vi "DAQ_Output TF.vi"(0 "System DAQ params to use:":u16(ring)=6 items=["MPS Rx", "MPS Tx", "Human Tx", "Rodent Tx", "Rodent Tx coupling (VRx)", "Rodent Rx", "Human Rx", "Manual Input"], 1 "TF_Params":T3={"Start freq (Hz)"=1000.0, "Stop freq (Hz)"=500000.0, "delta f (Hz)"=50.0, "samples per channel"=50000, "fsamp (Hz)"=2000000.0, "downsampling factor"=1.0, "Attenuation factor"=1.0} {"Start freq (Hz)" format="%#_6p"; "Stop freq (Hz)" format="%#_6p"; "delta f (Hz)" format="%#_6p"; "samples per channel" format="%.0p"; "fsamp (Hz)" format="%#_6p"; "downsampling factor" format="%#_6p"; "Attenuation factor" format="%#_6p"}, 2 "Save File?":bool=TRUE, 3 "string append to saved name":string="MPS_Tx_WithIMonNotch", 5 "Rogowski Scaling?":bool, 7 "Techron Gain Scaling":bool, 9 "Preamp Gain":dbl=1.0, 12 "User define frequency?":bool, 13 "Output all user defined value":bool, 14 "user defined \noutput value":dbl=0.1) -> (4 "TF mag output":dbl[](array[numeric])=[2.0372154916289125e-07, 6.793559181104437e-07, 1.696335790070309e-06, 2.1296488090751283e-06, 1.0109049448492243e-06, 3.242527142614195e-07, 2.01786175812527e-06, 1.3716083741435276e-06, 1.8749207637441033e-07, 5.690020511841858e-07, 1.3831526970474158e-06, 9.031002498074619e-07, 2.3120965479170196e-07, 4.2637533270188516e-07, 1.2717129807954672e-06, 6.739401216156862e-07, 9.502797117923468e-07, 1.4761926503177053e-06, 4.2449444146675436e-07, 1.3766268206166872e-06, 1.1574135065424225e-06, 4.390152066215787e-07, 1.4693364715610942e-07, 9.277841552509502e-07, 2.5102632307106685e-07, 1.5213042828718781e-06, 1.628993469736173e-06, 7.546981171721333e-07, 1.0427860563616102e-06, 9.714940189259299e-07, 1.43702270277105e-06, 1.2400316803756997e-06, 1.0637541376139376e-06, 7.466040945341502e-07, 8.974006467013478e-07, 3.6902682451535563e-07, 1.1637652293582506e-06, 6.6529859461445e-07, 1.5372963939506228e-06, 1.0372235089020587e-06, 1.3395277070635045e-06, 1.0361944250161835e-06, 1.3508414174132359e-06, 1.3622047310919937e-06, 1.0919652013386314e-06, 3.574766379241672e-07, 1.1659572050191398e-06, 6.189314025390137e-07, 1.0807867648715636e-07, 1.5380539400614782e-06, 1.6263735527414179e-06, 5.32112681526953e-07, 1.4310309890370497e-06, 1.4351885732615034e-06, 8.584318672907275e-07, 1.12233373437069e-06, 4.815228840574134e-07, 5.411977015167934e-07, 1.4144329557252704e-06, 1.1497955449729725e-06, 1.1095408290289881e-06, 9.59365615054982e-07, 1.8710766553428788e-06, 4.100069077682547e-07, 2.0252669578614933e-06, 2.0691205927940387e-06, 1.8891821441695545e-06, 2.0084794530702413e-06, 1.011117507818362e-06, 7.380670323609788e-07, 1.6387142491343077e-06, 9.327501315313441e-07, 1.8591321524715755e-06, 1.4227070668243068e-06, 2.6885456636705938e-06, 1.734732141488192e-06, 1.5359992596700657e-06, 2.9417755244459883e-06, 1.7998117427665506e-06, 1.2302735256347795e-06, 2.2271101093460748e-06, 2.0734509814401154e-06, 2.4002547859215057e-06, 1.4539712262088093e-06, 4.7436064752972777e-07, 1.882518473346791e-06, 2.9825459503646984e-06, 1.341447255240376e-06, 3.1473647714171137e-06, 2.401999152339036e-06, 3.830836392519218e-06, 2.7205751977305096e-06, 2.8678776825669147e-06, 3.3763181271312693e-06, 2.238606088769139e-06, 2.8006224623551447e-06, 4.226545237517427e-06, 3.936317527625128e-06, 3.5126357457397537e-06, 4.293951113248438e-06, 3.822800804203132e-06, 4.5225707303408105e-06, 4.0434439252313434e-06, 4.854193842370676e-06, 5.451288943225746e-06, 4.44612502569016e-06, 4.866573414449756e-06, 5.675666006001769e-06, 5.4403891145442125e-06, 5.75961684673854e-06, 4.870583216911151e-06, 6.4256941483989454e-06, 7.723671846367389e-06, 7.4837204474723845e-06, 6.222218548855555e-06, 7.590438086205701e-06, 7.5188758620780854e-06, 8.521498643916568e-06, 6.249152687634874e-06, 7.566289155689773e-06, 9.745623816846875e-06, 9.758296789658542e-06, 8.890595348675359e-06, 8.931120791337168e-06, 1.0399248680151127e-05, 1.0838503336982061e-05, 1.1260685540728752e-05, 1.082378468051051e-05, 1.2806779207580574e-05, 1.114960676394728e-05, 1.257128261917567e-05, 1.5416848441356857e-05, 1.4683523018574373e-05, 1.2611982709294083e-05, 1.642105662766135e-05, 1.5922423733550202e-05, 1.491421790154185e-05, 1.5578341427846582e-05, 1.659821358399733e-05, 1.709785681614034e-05, 1.8945273766490233e-05, 1.9363359923778153e-05, 1.9502597442375368e-05, 2.0639570485776163e-05, 2.0543207769782197e-05, 2.1691234755881526e-05, 2.2267028376064175e-05, 2.329089681548961e-05, 2.264594187261997e-05, 2.495996330527915e-05, 2.6105168892792582e-05, 2.7135537446387392e-05, 2.666988817069712e-05, 2.858416752662035e-05, 2.942859399006933e-05, 3.206928489966959e-05, 3.223048627196298e-05, 3.328739308435493e-05, 3.52415347598883e-05, 3.625643354079973e-05, 3.6778519243786124e-05, 3.811910848670486e-05, 3.90858476210099e-05, 4.221004792496587e-05, 4.22374549045834e-05, 4.5537077660884215e-05, 4.6308159049720095e-05, 4.878439550948665e-05, 4.9595461365732126e-05, 5.0734266319742015e-05, 5.335814071346675e-05, 5.617936948647044e-05, 5.7503826421850815e-05, 5.897541384195838e-05, 6.172515297231758e-05, 6.443664154470796e-05, 6.668646219152251e-05, 6.888677020126689e-05, 7.212234401398264e-05, 7.4933870118391e-05, 7.851452682634401e-05, 7.885553502658508e-05, 8.224084112024173e-05, 8.729351248339771e-05, 8.906874761983332e-05, 9.236254808123519e-05, 9.768310963065837e-05, 9.993873715919868e-05, 0.00010339897754066812, 0.00010898173400692462, 0.00011160171243173072, 0.00011706398053056314, 0.00012127098890446096, 0.00012650149142309162, 0.00013171434236989966, 0.00013758405099720852, 0.00014324117473233077, 0.00014863093132722968, 0.00015594197945553, 0.0001619041881869678, 0.00016946556001067674, 0.0001761666805086842, 0.00018437709377742338, 0.00019080859604449582, 0.00019887675407958386, 0.00020802928325185506, 0.00021735351743626773, 0.00022759683965656942, 0.00023772990243054828, 0.00024814096047077235, 0.0002577463712794448, 0.00026986599649594684, 0.00028340467395312254, 0.0002948052391906649, 0.00031149643710847764, 0.00032422266286623764, 0.00034155758920128947, 0.0003580001722440461, 0.00037535168678973295, 0.00039409138977495846, 0.00041430294696878433, 0.00043639323383142274, 0.0004607030690792594, 0.00048437378201234195, 0.0005116261720156887, 0.0005392744247378722, 0.0005716075743237706, 0.0006036990023538168, 0.0006382950959561843, 0.0006768368311226179, 0.0007184789659525549, 0.0007623862947976867, 0.0008130285347634719, 0.000865328852128615, 0.0009239292602682656, 0.0009882489296444742, 0.0010568390476129361, 0.0011338393422531956, 0.0012183921127213921, 0.0013138792442572388, 0.001418003747640743, 0.001535522947424366, 0.0016664493156874076, 0.001813297378252482, 0.0019799233643365286, 0.0021645534102197957, 0.0023784902298449747, 0.0026162768861308955, 0.002889733654480595, 0.0031963722989208, 0.0035374011016199606, 0.003914657200955006, 0.004323004729336459, 0.004753851195795146, 0.0051904836504763855, 0.005609851465877228, 0.005981794396312844, 0.006261726821948118, 0.00641179468539871, 0.006402195594109291, 0.006244408095304624, 0.00598702098189062, 0.005684764211770975, 0.005378027040291605, 0.005088639918349321, 0.004824671537009969, 0.004594773179979079, 0.004388250540076509, 0.0042074314116050835, 0.0040484671810071945, 0.003910154547206496, 0.0037847184253491078, 0.003676490229089884, 0.0035809616298052935, 0.0034950133528669955, 0.003419160313056956, 0.003355105939834968, 0.0032971154760109383, 0.0032458309179729584, 0.0032037401790805022, 0.003164161771550465, 0.0031327328175114557, 0.0031091482035021877, 0.003085498228113483, 0.0030690459185469996, 0.0030568044311039865, 0.0030461709143044836, 0.003041197505528879, 0.003041706349357348, 0.0030435455495283863, 0.0030495319370752966, 0.003057692641077951, 0.0030704250999599473, 0.0030849256090688644, 0.0031043793588513427, 0.0031261014737604203, 0.0031491108517110703, 0.0031771001385535913, 0.0032073608053417384, 0.0032436774293707585, 0.003279813325587537, 0.0033208704142117305, 0.0033637626362167028, 0.0034091342630075505, 0.0034592404274854695, 0.00351448277784265, 0.0035727253361016384, 0.0036334133511267274, 0.0036966059085619266, 0.003767518173210152, 0.0038413323284179116, 0.0039178981357463425, 0.004000713688535257, 0.004086254616971957, 0.0041774025214381645, 0.004274692122950266, 0.004374586450587849, 0.004480428652522378, 0.004592336922758399, 0.0047063586220150435, 0.004828329315829819, 0.004952304484767822, 0.005083864418425228, 0.005219992544257958, 0.005360572150230163, 0.005503310775577753, 0.005650178099919648, 0.005797876043917457, 0.005947310317132557, 0.00609322438643053, 0.006240068116715204, 0.006381286601970306, 0.0065199452791355975, 0.006648805426228001, 0.006764667255400801, 0.00687148605986856, 0.0069620532378664385, 0.007034500737286003, 0.007088490320480461, 0.007123016978728839, 0.007135629768528894, 0.0071272667489462455, 0.007097935162051244, 0.00704688833896544, 0.00698063251987629, 0.0068993456960810325, 0.0068020652511235295, 0.006690301151635434, 0.006572939495142656, 0.006445477583369852, 0.006313942018104493, 0.006176322525557588, 0.006042932950458157, 0.0059062422568806885, 0.005759142682368877, 0.005619395191586785, 0.005500699809907893, 0.0053677371581780774, 0.005240933031342609, 0.005116506843688415, 0.004997998143370529, 0.004882573974520269, 0.0047699918897461824, 0.0046653540271694065, 0.00456423216909828, 0.004465264326574151, 0.004374492456427474, 0.004285528727967664, 0.004199866013002946, 0.004117968553655641, 0.004042080261713175, 0.0039676189128161595, 0.0038954429953121715, 0.003829986170977068, 0.0037660919612099294, 0.0037041343225806614, 0.0036459363198869895, 0.003590625647267971, 0.0035373602829234093, 0.0034856488342473882, 0.0034397914012131714, 0.0033936480297744203, 0.003349844232891371, 0.0033070063257520676, 0.003270540153728508, 0.003232013758206085, 0.0031971683916848528, 0.003164100942299467, 0.003132074968409261, 0.003102906016181999, 0.0030749530093250694, 0.003048557411793342, 0.0030251150856024337, 0.003001299830241231, 0.0029798512534916447, 0.0029588722539942622, 0.0029426250122048113, 0.0029261826415382143, 0.0029099037261367143, 0.002897980720198404, 0.00288340882160916, 0.002874341499206318, 0.0028661737074489224, 0.002857012307988124, 0.0028517467867249452, 0.002849270969549165, 0.0028426491181320385, 0.002843598198764933, 0.0028456501701090817, 0.002846987016539148, 0.0028546148348877858, 0.002861468125705527, 0.0028696341944694655, 0.0028821643213220263, 0.0028958483242476148, 0.0029124092621891392, 0.002932028600726075, 0.002955969060847836, 0.0029808809710248755, 0.00301074312654329, 0.003044911212316796, 0.003086668441052093, 0.003123561677421555, 0.003177631079607654, 0.003220900345320899, 0.003283404786445936, 0.0033335077077304505, 0.003415158770545732, 0.0034917469944288613, 0.003574823389508343, 0.0036591756984979628, 0.0037449425633328494, 0.0038316979794502395, 0.003908487950184218, 0.003968842309478478, 0.004003554932827288, 0.004000305003242141, 0.003944326724562689, 0.0038282707078578357, 0.0036551095435839055, 0.003430591002762993, 0.0031729199038966985, 0.002897570133363583, 0.0026221348457451253, 0.0023620070095678857, 6.164614697188743e-07, 0.0019030029843609476, 0.0017124606132191383, 0.0015463391035798878, 0.0014045425244661302, 0.001283156041583334, 0.0011783872907193238, 0.0011062852186959325, 0.0010345130604953571, 0.0009862645351283305, 0.000951913213045555, 0.000930822971927366, 0.0009229063773060129, 0.0009278401171160928, 0.000947666169095748, 0.0009782281520481502, 0.0010238234384319386, 0.0010867909292265497, 0.0011655078777641108, 0.0012626822383428405, 0.0013807053346902112, 0.001518885518425445, 0.0016807681781777079, 0.0018709546877245882, 0.0020858300920659273, 0.002328247444811447, 0.0025927272793475984, 0.0028785096374129744, 0.0031688479973878093, 0.003448477146808804, 0.003703943351999831, 0.003916319650435753, 0.004072372564256995, 0.004174102273354721, 0.004222381703749427, 0.004228257581942058, 0.004198666137537497, 0.004150743924274754, 0.004089118026205858, 0.00402012832415787, 0.003953650143401563, 0.0038847672330356367, 0.003820782968838551, 0.0037626870141772508, 0.003705343736908736, 0.003658006130046551, 0.003614856738190562, 0.0035784208320527515, 0.0035434238584049283, 0.003514160478534067, 0.003488170700812893, 0.003468622707332244, 0.003443915344896603, 0.0034314299162463134, 0.0034246630437881663, 0.003416544978817137, 0.0034119641099697425, 0.0034088364558863206, 0.0034083014897694965, 0.0034117155961883717, 0.0034159402473708006, 0.0034217779007516633, 0.003430072444593314, 0.003440049913353305, 0.0034538917831024966, 0.0034669055423229133, 0.0034833364863646864, 0.003501628475332639, 0.0035196197032543912, 0.003540336254543647, 0.0035622786880641732, 0.003585694628045036, 0.003611895491815887, 0.003640008384025932, 0.003667157114489658, 0.003696788673689253, 0.0037309122101256507, 0.003762746847704778, 0.0037970057968524425, 0.0038353516289641766, 0.0038714577040932846, 0.0039113841049076715, 0.00395147652947973, 0.003995491778150964, 0.00403812158458586, 0.004087585217075255, 0.004134714990345707, 0.004184749090863663, 0.004237536259964986, 0.004289462606464673, 0.004345586835427315, 0.004404102710112459, 0.004463315212311432, 0.004525851738043004, 0.004588374389625155, 0.004657469223876116, 0.00472500859303859, 0.0047969494885303195, 0.00487141632955198, 0.004947756733803814, 0.005026829427225351, 0.005108658634518159, 0.005194617350463291, 0.00528248025974792, 0.005371866803911184, 0.005466752222299172, 0.005562387013028619, 0.00566560323632966, 0.005767577425601827, 0.00587687501776066, 0.005987009019026231, 0.006102088996437571, 0.006223627687271268, 0.006345229034043439, 0.00647128049002447, 0.006605011436205142, 0.006739802231268402, 0.0068799279793823566, 0.007024819960270474, 0.0071753374378373215, 0.007327972898878207, 0.0074888643285302555, 0.0076499912263523805, 0.00781978907948591, 0.007994419869134756, 0.00817024970975524, 0.008349410641485283, 0.008535727849152727, 0.008723027999915828, 0.008916179810292683, 0.009110973170224202, 0.009310867548075983, 0.00951180121726737, 0.009711672504489894, 0.009913334696390445, 0.010112796222984012, 0.01031388040365655, 0.010512437920119903, 0.010704567828247245, 0.010895515977437925, 0.011074623324110815, 0.011248750272778663, 0.011411509034678248, 0.011562649968872745, 0.011701942061589638, 0.011832798950041565, 0.011940517202510381, 0.012037413785487755, 0.012114521830438083, 0.012174924860481079, 0.012216767323894755, 0.012243209207602959, 0.012247709617285987, 0.012240010247821648, 0.012209836313097716, 0.012168028995498176, 0.012109759173068004, 0.012034522182703776, 0.011948772525407365, 0.011851525989082679, 0.011745454590657902, 0.011628240665402894, 0.011505038496599857, 0.011376852844174962, 0.011239735443193379, 0.011103832677707079, 0.010962850555773767, 0.010822065607391079, 0.010680625672971084, 0.010535385013054266, 0.01039054769482169, 0.01025176171211727, 0.010113251395753366, 0.009971691355567611, 0.009834262067813083, 0.009702255710372124, 0.009574029455887891, 0.009446822900503322, 0.009319720522908803, 0.009201529228534809, 0.009082694467120624, 0.008971962377477155, 0.008861154816449937, 0.008756517789594447, 0.008653410153402935, 0.00855409504766486, 0.008457961508651883, 0.008367952582596505, 0.008278244688673891, 0.008192999415495356, 0.008111552392976442, 0.008036794780504616, 0.00796144879230125, 0.007888979685585542, 0.007819344480339802, 0.007754288285094333, 0.007694339832065249, 0.007634104724108179, 0.007575291221359333, 0.007522567947202587, 0.007469221398234218, 0.007423758302493742, 0.007378140377463572, 0.007335127075570248, 0.007292968067296177, 0.007259098778388161, 0.007222119021201777, 0.007190322865531502, 0.007160372613883688, 0.0071328789176969744, 0.007106856861104297, 0.007086815067238445, 0.007065491821345224, 5.546838338613242e-07, 0.007031486378227067, 0.007019384683356254, 0.007010062760928216, 0.007000077530297156, 0.006995370883301304, 0.006991647291921397, 0.006990644822433608, 0.006991325452510118, 0.006995689108552698, 0.0070002833959157745, 0.007008318610279569, 0.007021193674572225, 0.007032760654437141, 0.00704952640215466, 0.007068003637619281, 0.007090315730289243, 0.007111636934614471, 0.007141592610911906, 0.0071683670064617636, 0.007201021141207065, 0.007236459974853032, 0.007277386141220549, 0.007316987402201348, 0.007363517240918104, 0.007409807563783298, 0.007462479587681477, 0.007518549491041108, 0.007576989843540695, 0.007636498399831262, 0.007705430767937352, 0.007778317588309633, 0.007852434050960916, 0.007929901774595809, 0.008015542942976071, 0.008103912510163734, 0.008200019508343339, 0.008296823702025974, 0.008406222769244142, 0.008514706615279491, 0.008636830705876924, 0.008758847294239562, 0.008894024140768399, 0.009032297369439196, 0.009181338441392796, 0.009326957459033012, 0.009501365304138455, 0.009674120938744847, 0.009859894704024064, 0.010053693985701787, 0.010259551491084148, 0.010479289260633656, 0.010707560752033028, 0.01095149664420516, 0.011210562391792548, 0.011486347046830546, 0.01177137799579019, 0.012073752819968331, 0.012395791965619964, 0.012729353691860342, 0.013089748942432861, 0.013460368571250637, 0.01385977342398694, 0.014265912195477652, 0.014697306686528744, 0.01514034539102792, 0.01560757849564455, 0.016075815847262413, 0.016564786538784054, 0.01704467463433095, 0.017533088951704023, 0.018015748889576716, 0.018475590459784356, 0.01889974690987198, 0.01930318427234332, 0.01964640577240411, 0.019925382568646396, 0.020228750568243768, 0.020265656705801476, 0.020297101520647225, 0.02024819226764239, 0.020098609687792555, 0.019856752080114056, 0.01953181759374221, 0.019144129055940963, 0.01867901461616855, 0.018180542030335513, 0.017641175407968206, 0.017085042585021932, 0.01651585903499849, 0.015949546801429192, 0.015382417645858707, 0.014834707677971133, 0.014296118869649967, 0.013782714967972598, 0.013282214801240469, 0.012811679509594128, 0.01235581070612155, 0.011927878790376219, 0.011519248800922687, 0.011127343542270155, 0.010752867280692132, 0.010411375755346888, 0.010078041405944737, 0.009767792276147947, 0.00947034287789845, 0.009191394000659462, 0.008924938111006048, 0.00867416964508942, 0.008435748159650501, 0.008211731744829516, 0.00799628612106185, 0.007798892356861463, 0.007602257981305233, 0.007423579551743067, 0.007249260954099596, 0.007087197639072701, 0.006930931211151319, 0.006786447695694304, 0.006643871181243099, 0.006511490766310069, 0.006385141774894306, 0.006267532596712949, 0.0061546566403550725, 0.006047018999790388, 0.005941378993852128, 0.00584868739064578, 0.0057546480814531795, 0.005667347668829675, 0.005586641463647396, 0.005508203587509282, 0.005433859524928404, 0.0053663009906424666, 0.005303500780531138, 0.005237420541909372, 0.0051812790486258035, 0.005127022459714558, 0.005075951477162811, 0.005030904536023909, 0.004986705805615258, 0.0049495604105589345, 0.004911452237008161, 0.004878000151050528, 0.004848643960764925, 0.004820642274108188, 0.004798972787378096, 0.004778082269931038, 0.00476188171304398, 0.004747220842243101, 0.0047354648145581085, 0.004727605176166839, 0.0047231266040788575, 0.004723463322165673, 0.0047234203044524145, 0.004729862440449979, 0.004738910028400524, 0.004751708118108957, 0.00476396834240096, 0.0047829184196307205, 0.004804059455298296, 0.004826942512691633, 0.004854623108493706, 0.004883439403248536, 0.004918143878170193, 0.004951495940519052, 0.004986553952624207, 0.005024245245054637, 0.005062482316529173, 0.005096471034425928, 0.005128313819767421, 0.005160779122739624, 0.005187588441927762, 0.00520399372392812, 0.005211739706816874, 0.005209051196474495, 0.005194689792525376, 0.005162054410679822, 0.005113774627149544, 0.005046082674903037, 0.004959945257122816, 0.0048543749246190955, 0.0047262901579443175, 0.004588743282303231, 0.004433977168555782, 0.004267307407971839, 0.004090938607897501, 0.00391167568652165, 0.003728920388539005, 0.003543671676833687, 0.0033621656039902314, 0.0031853263396406034, 0.00301245296775813, 0.0028467892137657045, 0.0026879681915949784, 0.002537911379031695, 0.0023958245784159106, 0.0022605598807129506, 0.002131527399077782, 0.002013108429582286, 0.0018994132677840946, 0.0017943346889407246, 0.0016936111510475094, 0.001600469525632794, 0.0015115940886708712, 0.0014304339331459414, 0.001353339985544366, 0.0012777062666591889, 0.0012195131974909242, 0.0011379246097210683, 0.0010883136080910775, 0.0010313189156855105, 0.0009771522811846648, 0.0009286224642889719, 0.0008808977562469889, 0.0008359982858023881, 0.0007947717424571735, 0.0007548929610178948, 0.000717501683787555, 0.000681324549907791, 0.0006467839458602313, 0.0006200034438237885, 0.0005883191937759186, 0.0005601993506408708, 0.0005313376620691447, 0.0005063887690977925, 0.00048202868815941505, 0.00045916625487411763, 0.00043809039057423347, 0.0004167681990561311, 0.0003972543806660549, 0.0003783056441678319, 0.00036183135494363103, 0.0003438086130131863, 0.0003285076928817975, 0.0003135112552121596, 0.00029902740610936624, 0.000285022946143483, 0.0002717845781508606, 0.00025846023178235006, 0.00024778789406428167, 0.00023657754203818424, 0.00022332645406769833, 0.0002130844148469932, 0.00020518906409604145, 0.00019495229220741514, 0.0001868515457089178, 0.00017666430828974322, 0.00016945486922525382, 0.00016173597016781155, 0.00015427290194259987, 0.00014583017928042558, 0.0001394532040387906, 0.0001324241771500869, 0.0001280933345118669, 0.00012156619509743325, 0.00011824407941880821, 0.00011236776242865911, 0.00010624416956535214, 0.0001027357132786282, 9.92123558802412e-05, 9.197764102919613e-05, 8.931515920821514e-05, 8.719661434611681e-05, 8.244250929818397e-05, 7.94297083637959e-05, 7.813929467799097e-05, 7.603798394004373e-05, 7.350762399698821e-05, 7.12151393165494e-05, 6.895482838131393e-05, 6.671046611850901e-05, 6.407147910490223e-05, 6.389699746887125e-05, 6.247957839954287e-05, 6.289629989829454e-05, 6.194387743455696e-05, 6.135465502450149e-05, 6.087816993385767e-05, 5.816000315461685e-05, 5.923397859448671e-05, 5.86711645637256e-05, 5.863345428538828e-05, 6.070839663391591e-05, 6.0338799568149135e-05, 6.015464172175751e-05, 5.9917620265870535e-05, 5.959781431737995e-05, 6.0454716706029717e-05, 6.063455580839131e-05, 6.009608800981641e-05, 6.387706217422418e-05, 6.34600791090772e-05, 6.431548066813142e-05, 6.457014794584466e-05, 6.593560505304135e-05, 6.4601604384995e-05, 6.63249236881072e-05, 6.604359174471053e-05, 6.675061933962089e-05, 6.713102039404873e-05, 6.681963999985778e-05, 6.768736972693942e-05, 6.9183790534655e-05, 6.942822624230465e-05, 6.982843956190732e-05, 7.193672496854038e-05, 7.021436074452037e-05, 7.17975311597413e-05, 7.183611942498269e-05, 7.012259519525509e-05, 7.377322279735478e-05, 7.29699143899538e-05, 7.204364394322717e-05, 7.43419969560943e-05, 7.469514547335262e-05, 7.474792352170519e-05, 7.535147016489018e-05, 7.588840885577198e-05, 7.640960372794765e-05, 7.489888720309596e-05, 7.603121348222829e-05, 7.723520923735244e-05, 7.716898340179197e-05, 7.879828943663293e-05, 7.878918964207931e-05, 7.839321345408815e-05, 8.067898332242799e-05, 8.023573677573643e-05, 7.933387960652674e-05, 7.879289310481334e-05, 8.083210121646043e-05, 7.918232639055638e-05, 8.120955801247514e-05, 7.963947724208541e-05, 8.232498935875233e-05, 8.05674053536353e-05, 8.18622968308476e-05, 8.207496156961378e-05, 8.15947348367063e-05, 8.124371368542347e-05, 8.220147361838506e-05, 8.33574764778626e-05, 8.242382265869806e-05, 8.365398123681995e-05, 8.293297779392434e-05, 8.439847730918912e-05, 8.368439680869435e-05, 8.363405707304298e-05, 8.384303639641865e-05, 8.422979774229118e-05, 8.364030257485974e-05, 8.403107482227207e-05, 8.367083835093945e-05, 8.41160485051156e-05, 8.531238157073731e-05, 8.508144025133058e-05, 8.590405766901755e-05, 8.477426803288628e-05, 8.543434513154186e-05, 8.533576780752976e-05, 8.659463549318744e-05, 8.535511698671412e-05, 8.613472455143942e-05, 8.490919102595647e-05, 8.625111789073192e-05, 8.635640454191086e-05, 8.698594769204356e-05, 8.6389368874127e-05, 8.61667281379288e-05, 8.64699495096001e-05, 8.595826222889964e-05, 8.723248182699668e-05, 8.64711328992852e-05, 8.693144214833651e-05, 8.683641652517674e-05, 8.78958393738193e-05, 8.734492345960697e-05, 8.783916049823444e-05, 8.61747002264401e-05, 8.768501804301456e-05, 8.714337518653518e-05, 8.747270502178725e-05, 8.750948775232275e-05, 8.74785819433097e-05, 8.792969324249523e-05, 8.73497058898647e-05, 8.930668794129315e-05, 8.779903464005035e-05, 8.828630900858057e-05, 8.889849288226898e-05, 8.855524954678201e-05, 8.964311602247672e-05, 8.810725925489338e-05, 8.962789018095396e-05, 9.014890836021389e-05, 8.915746994358566e-05, 8.930245017529432e-05, 8.878742269477327e-05, 8.940407714523939e-05, 8.968701613923263e-05, 9.088473137324469e-05, 9.027823306624076e-05, 8.977618841059141e-05, 9.012271611846928e-05, 9.057658169548787e-05, 9.15894221167761e-05, 9.028928117230089e-05, 9.063918569159491e-05, 9.25414067258851e-05, 9.298417304110964e-05, 9.134810452844022e-05, 9.190862191879943e-05, 9.339926616916888e-05, 9.212173087654502e-05, 9.246865273698261e-05, 9.306556468780206e-05, 9.303785247470485e-05, 9.277106558924882e-05, 9.192346456547312e-05, 9.262687474891765e-05, 9.330804877002039e-05, 9.30915387511946e-05, 9.38819292239803e-05, 9.543702349636271e-05, 9.560762127592522e-05, 9.508206330111681e-05, 9.5773149779388e-05, 9.608461691968223e-05, 9.731825843248855e-05, 9.537184511560309e-05, 9.54180350620616e-05, 9.679352690109114e-05, 9.732014345971237e-05, 9.813862006561962e-05, 9.775702394087522e-05, 9.849364337657339e-05, 9.829811450182467e-05, 0.00010056198340261321, 9.948285592328476e-05, 0.0001012267969665088, 0.00010026707751442345, 0.00010103461637476879, 0.0001019729753169905, 0.0001023362558214886, 0.00010247887907697833, 0.00010374506914512854, 0.00010197042681756403, 0.00010476583496666581, 0.00010325909274254808, 0.00010629689913288521, 0.00010782386048494457, 0.00010741281145145474, 0.00010785649671445314, 0.00010796738992431124, 0.00010777079182075159, 0.00010921659144371598, 0.00010943866598092394, 0.00011146174333304786, 0.00011084242318885517, 0.00011197824630743252, 0.00011340437595824194, 0.00011272829548002021, 0.00011505593396547745, 0.00011541774570122776, 0.00011616030536194512, 0.00011929865636628787, 0.00011825591447429914, 0.00011955326898795407, 0.00011995860152418436, 0.00012092833277953469, 0.00012270402817089008, 0.00012425441117186207, 0.0001245517907204726, 0.00012645246589899697, 0.00012797859413697687, 0.00012933765190669097, 0.00013037304046320918, 0.00013189593423435948, 0.00013374897228205984, 0.00013426913231691468, 0.00013686423148932193, 0.00013880149350947122, 0.00014026492531460285, 0.00014126619942793188, 0.00014469672761256467, 0.0001451596187744496, 0.00014609905755956138, 0.0001477942496824828, 0.00015133777868834273, 0.00015267119910958145, 0.00015498770227151035, 0.00015604023917850386, 0.00015965494152595224, 0.0001622110708458638, 0.0001648701780762397, 0.00016733902867963459, 0.00016860833373585278, 0.00017078227504466374, 0.0001739919117484125, 0.00017568680941388613, 0.0001791747440530861, 0.0001807124287897092, 0.0001837401329950777, 0.00018540067962826917, 0.000186033485964296, 0.0001895892756066794, 0.00018949324593250016, 0.0001932350189542062, 0.0001944399181849291, 0.00019674787263664647, 0.0001946885378691641, 0.000197202418587247, 0.0001990327346228414, 0.00020013533937909427, 0.00019980851055136233, 0.00019745364056866606, 0.00019663877453312357, 0.0001953699001856613, 0.00019446932804834517, 0.0001916928082036627, 0.00018950173913956616, 0.00018802891860576486, 0.00018442938484860804], 6 "TF phase output":dbl[](array[numeric])=[-2.8411090470349776, 1.5669503825450217, -1.1478587631654162, -2.133303992553073, -1.6508550639764503, 0.14003797314127198, 2.784849537654816, 2.1929890555943596, -1.3836048892463826, -0.8769344037550304, 2.8272489837633685, -0.1467449692789624, 0.8726462407001185, -2.5250218357801995, 1.7366075027402315, 1.5087137147136493, -2.3229837034753213, 1.9373201006639098, -1.363740091299091, 0.5435556977044127, -3.066135316068815, 1.7590880940434408, -0.8082243792779371, -0.0769197320187025, 2.088501718638536, -2.654159790462069, 1.1352494061642724, 0.6903120997194957, -1.459915191985042, -2.9543137518264087, -2.9912729384528607, 2.3168381770215363, 0.2616382563523534, 0.19461451861802728, 2.781663361521798, -2.809510779433071, -3.118732667348869, 0.13482044140709126, -2.1396548384508196, -2.776645338015605, 3.0972385485480673, 0.7407336336309752, -2.6315828971861643, 1.3130682193432206, 0.14948071647419292, -2.431287862741484, -1.0828884031114054, 0.4578917043109607, 2.6302833965125396, 2.5589678024387426, -1.8776911658383855, 3.015562814496311, -2.1128760344004025, 2.8398750977887848, -2.2232313092442633, 2.663902298952091, 2.778409180981473, 2.530953023596568, 1.145713909247232, -3.0687691231831304, -2.8023159311724446, 1.9061425258675286, 3.006358400933046, 2.759392376736137, -2.4984973147070075, 2.712559247608158, 2.8893171685740886, -2.0044541564833738, 2.7699982150716034, 0.16930625597387078, 3.06581231079713, 0.6779385160089745, -2.6692875859457765, -2.476398150450236, -3.08997955159424, 2.7600413613817496, -2.799888453285187, -2.7941269406303633, 2.8288704568899683, 2.9730778025568223, -2.7913826980820473, -2.5945772145442083, -3.1066341814309677, -3.074234521246678, -1.5809575638116025, -2.5121738830867315, -3.0283590465598094, -2.8754989108165825, -2.9182916505864545, 3.0270458128788142, 2.9942961108065855, 3.037009649286636, 2.882586942488975, -3.070864948213993, -2.9961199198175463, -2.689193244342652, -3.0468519796340847, -2.976369057478769, 2.8159643621635286, -3.0786940188619942, -2.8913714626407936, -3.042761831249641, 3.140335103077841, -2.984198472733842, 3.079838424409013, 3.0193495561616768, 3.0608960943475885, -3.1011373035704946, 3.0033986514532853, 2.836867844269223, -3.111450011571117, 2.9509804659502703, 2.992104602760614, 3.1116164726799203, -3.1109028082406502, -3.042382762821636, -3.0938137422617964, 3.090248902262086, 2.978096891986455, 2.903071601960301, 3.065032774030024, 3.0147759959126437, 3.0311678576917416, 3.046554836254789, 3.0034940353918342, 3.085484360153145, 3.0272503203731347, 3.083105086700099, 3.0865690148745486, 3.084887354757639, 2.8818946862674046, 2.9974487116938233, 3.0132397611529718, 3.0014522872055633, 2.9804960247370516, 3.0322207222930486, 3.1096429552172045, 2.967951496352894, 3.025974852340799, -3.0239560048742686, 3.0215906260747283, 3.0814734514988116, 3.034181437759039, 3.0408167294408868, 3.024265872940204, 3.0603992114904246, 3.0306794774441745, 3.055569522097212, 3.023701050120206, 3.0163261616460875, 3.037641291907729, 3.0677335460837045, 3.0216958876032165, 3.04002905825061, 2.989479140078021, 2.980610711285365, 3.012166487262641, 3.0496943743594818, 3.030417189477702, 3.035257318229471, 2.9913973990011073, 3.057220230453412, 3.0466495206440634, 3.016422403948623, 3.006004992663699, 3.016710513715707, 2.9845942802914416, 3.012937817859491, 3.015913947242596, 3.023422656698271, 2.9916980011595604, 3.005209789534568, 3.004932686844181, 2.99303854059888, 2.974937195945119, 2.9887611211664664, 2.973491478514034, 2.9675983633919283, 2.9900160393417585, 2.9639639015604895, 2.9825515184072544, 2.9754358597308954, 2.9736152136641176, 2.963114534606136, 2.96993126764279, 2.976715269057363, 2.9774636018690357, 2.9607266651774746, 2.9580107390431687, 2.9554784448478744, 2.9581978647658373, 2.9558635066559886, 2.950825570841959, 2.9657988900127283, 2.9425260441042176, 2.9352022489825402, 2.9425891112958036, 2.9363968380689207, 2.944550049744829, 2.9270433218571403, 2.931044103562728, 2.9206848032780215, 2.9223202436822193, 2.9267494026161667, 2.9170438332330764, 2.9131791325922776, 2.9052814921859715, 2.9006234294113864, 2.90133533517305, 2.8971561212936803, 2.893827979170931, 2.8969195303199933, 2.8845573550635772, 2.8823324467712044, 2.8785101552622003, 2.872430981832738, 2.866810736690213, 2.8672434967758993, 2.8591259858275135, 2.849459872294885, 2.844302430091522, 2.838413465932962, 2.8335586850778642, 2.825330533986348, 2.8202276776016353, 2.8118288450916475, 2.805444308972642, 2.7976593858595713, 2.785442064554154, 2.777860033483804, 2.7680015572352095, 2.7579958748494624, 2.74592825262836, 2.7347593754022377, 2.723035155844549, 2.7104387997314614, 2.696527443600788, 2.681310326593861, 2.6636619530570527, 2.6440334087498827, 2.6226207897389853, 2.60095077458205, 2.5762898140296384, 2.5468010681431568, 2.516138096346058, 2.4805245824447457, 2.4402173087913708, 2.395234588367308, 2.342256046878575, 2.2825924230668906, 2.2139537001239664, 2.1371168877895768, 2.0476183758915676, 1.947312755471584, 1.833977306603648, 1.7072820842586915, 1.5668020329177188, 1.4153402610484809, 1.2537734598629195, 1.0901257790194876, 0.9330171988885464, 0.7922941553709885, 0.6723793677254981, 0.570628534510435, 0.48597973329592437, 0.4141078977217245, 0.35285656554312966, 0.3000945527859564, 0.25430042697093896, 0.21362105960625152, 0.17811568955642043, 0.14626680997477304, 0.11610583819114148, 0.09029005444551744, 0.06590384890571954, 0.04338519998702873, 0.02248770116385358, 0.0027534456457267834, -0.014788863668160148, -0.03246402392973755, -0.04866248190247479, -0.06391194759906128, -0.07919984379285164, -0.09345600106796235, -0.10798458157637647, -0.12119822608432651, -0.1348274737854334, -0.1472056923710696, -0.1595612353270588, -0.17193917893055624, -0.18473113948460315, -0.19678452977680627, -0.2083908175952229, -0.22056548602165618, -0.23316514999105856, -0.24463158821978073, -0.2574303199797745, -0.2701503695787894, -0.2820737000642688, -0.2949288403312909, -0.30790895630348863, -0.3216085728414096, -0.33443364039144563, -0.3490199415269901, -0.3623873104173698, -0.3769038336898968, -0.39248420224709085, -0.407384484213724, -0.4231518175538571, -0.4401444158312782, -0.45724511043126864, -0.4744297709897176, -0.49285146039811506, -0.5118692013907934, -0.5321874153778732, -0.5532505989727476, -0.5757979884253792, -0.5986954801146358, -0.6227055473644424, -0.6478670484401747, -0.6741173149072888, -0.7019526358181015, -0.730735813470847, -0.7627488024814223, -0.7939535341402679, -0.8293331082878674, -0.8650051139139819, -0.903033124196873, -0.9430913325136183, -0.9842254193894717, -1.028313116148226, -1.073460918358514, -1.1213070900925406, -1.1709614868819476, -1.222076510478047, -1.2762697358097261, -1.3295992801229244, -1.3850369442454982, -1.442130072091561, -1.4984988154787173, -1.5559120274400577, -1.6117169251858283, -1.6677355245496015, -1.7244561936458571, -1.7781124029832212, -1.8308198077503333, -1.882377771708138, -1.9318932655971697, -1.9798817272895237, -2.024792404049358, -2.0676311896919217, -2.1105781399669734, -2.1505415608340446, -2.1878502468182996, -2.2220671880145177, -2.2554361470157556, -2.2884789849990335, -2.3194072240342876, -2.3464137922619237, -2.3732308413776195, -2.398503287980774, -2.4236074210171177, -2.445832366003324, -2.468642271633127, -2.488736724926318, -2.5079191456726773, -2.5269117852835126, -2.544271896856939, -2.560788859592762, -2.576269067852534, -2.5917256282875782, -2.606872405202708, -2.6200894052799435, -2.6323614075401287, -2.6453888408229154, -2.657509104981763, -2.6687258646066128, -2.680295397654868, -2.690940641087754, -2.7010947757695494, -2.708678357854751, -2.7179518048561877, -2.7271789408638774, -2.736166230410929, -2.7440831959714185, -2.7517095938233145, -2.7596800456923005, -2.7671539757236405, -2.77323506864739, -2.779734608757077, -2.787193038464296, -2.7934668796203455, -2.7989904509879375, -2.804789733390986, -2.8098045119020663, -2.8160954148786526, -2.821344741443378, -2.825937963053795, -2.8305757702120338, -2.836471904558297, -2.8408750952179527, -2.8457152003321204, -2.8502642587785236, -2.853970236982018, -2.8585704661226523, -2.8625603358573324, -2.867400392985319, -2.8716964882000933, -2.8768179813828056, -2.881609230907792, -2.8857229720153192, -2.8904405835862828, -2.8940289030647177, -2.900666532853601, -2.9056907968669656, -2.9109087342591797, -2.9173406194767133, -2.9232934813629687, -2.9302376158743235, -2.9377212379377946, -2.947126832678916, -2.9556079410968374, -2.9666030035040447, -2.9783770238435183, -2.9925776762375973, -3.0089494101185528, -3.027514884862243, -3.0482016438747985, -3.073270708421855, -3.102770939244396, -3.1366189800816393, 3.1064784405012946, 3.059564871292909, 3.0040263903007074, 2.9407220832432444, 2.8689599977435813, 2.789921555981138, 2.7043892379959478, 2.6156106823658627, 2.5279992988764177, 2.447263185522248, 2.3759440018499425, 2.3159388775592027, 2.271997112658157, 2.2452785791281396, -0.3488542054903079, 2.236691858078724, 2.254971270857029, 2.2867735252187544, 2.33139476008575, 2.389439157626549, 2.4575408517405015, 2.528236227387926, 2.625521115012923, 2.7187659142680713, 2.8188387949364384, 2.9240464631161984, 3.0300747923173774, 3.135163227686434, -3.042137838447917, -2.9383324429787163, -2.8430280068796225, -2.752971691741129, -2.6714194477385087, -2.5976682867673224, -2.535286453506132, -2.4861067190272492, -2.4508379299542864, -2.424871225666465, -2.416113692639799, -2.420959873539099, -2.4420615547915023, -2.4781134075576645, -2.529946522657997, -2.594300664571784, -2.669323426433799, -2.7505568204469846, -2.8350822478260183, -2.9170212543583482, -2.99571360832986, -3.065548474636341, -3.128522496802789, 3.0986729998449682, 3.051676532342239, 3.0100561708406572, 2.9740637576739193, 2.9444378850200605, 2.9197684873376875, 2.896951990598756, 2.8789684701379326, 2.8623894113244823, 2.8483124096992496, 2.835633468110231, 2.824798952910446, 2.8138641606365633, 2.805671724874828, 2.7976415560320467, 2.7898806158737965, 2.7868591616813085, 2.7759583009162316, 2.775139947359887, 2.7689882997567117, 2.765209757776232, 2.759979559389761, 2.755890823286421, 2.7526373975030496, 2.7485449775993636, 2.7434870862891723, 2.7410619914307084, 2.7366612875451595, 2.7335642217249387, 2.7305850397418263, 2.7261449823998776, 2.7240612125156956, 2.7203639672933972, 2.716421168404425, 2.7110474592337175, 2.7080888087941606, 2.704835983567937, 2.6999921826379674, 2.6960572437376134, 2.692162714458271, 2.68841910002532, 2.68382481804715, 2.68042236199599, 2.6746332198461467, 2.6695973019255144, 2.66557223993584, 2.6604504335589136, 2.6548082693699198, 2.6500053162299086, 2.6453229082487186, 2.6398673064488656, 2.6332120815135642, 2.627553718123872, 2.622093539075034, 2.614741858871235, 2.6098790471873716, 2.6020911513003133, 2.5968457304883072, 2.588820887481173, 2.580757785372984, 2.573898140112586, 2.5662812567998206, 2.558454633507633, 2.5504420854415066, 2.541441937972475, 2.532519122379549, 2.5233686507782407, 2.514771804398488, 2.503832176500931, 2.4938403016177046, 2.4838790831035467, 2.473128959254347, 2.4615717080979143, 2.4490329679334915, 2.4373905470127424, 2.425336213279914, 2.411642401071607, 2.3985233059865863, 2.3833120033934514, 2.3692510726653824, 2.3530803992986677, 2.338211657035387, 2.3226470777890498, 2.3046379141061486, 2.2861452643683506, 2.267890939741732, 2.2485223938421046, 2.2294220718220763, 2.208191101836067, 2.1865622645598575, 2.1648171414318997, 2.1403372927389235, 2.1174663218052627, 2.0922550191576437, 2.065558261671758, 2.0376278546823894, 2.0102126286949202, 1.9802275181330884, 1.9511682016506664, 1.9187162728501437, 1.8861388068817038, 1.8538711806023016, 1.8190652209808562, 1.7829834340165251, 1.7482773497559494, 1.7097955133094696, 1.671825542450362, 1.6333777141433956, 1.5947598185849585, 1.555360523812295, 1.515709279717564, 1.4750508221916951, 1.4352625391572604, 1.39517379389802, 1.3542468546589823, 1.3132852240404702, 1.2740393789126905, 1.2346461880436836, 1.1956734202290262, 1.1564214745447425, 1.1205462651448461, 1.0824966654037478, 1.0474425882687608, 1.0124407116133312, 0.9780215186249543, 0.9459251042972756, 0.912380724822225, 0.8830965757117142, 0.8522026523607705, 0.8236038048481826, 0.7958710170156053, 0.7672858420074975, 0.7418338484475167, 0.7162014749231622, 0.6920162072078558, 0.6683360260464686, 0.6479176478685787, 0.6248336650499653, 0.6040408747605645, 0.5840952189553681, 0.5637128049809225, 0.5454301068305389, 0.5282745158313509, 0.509646710199768, 0.4936445024058767, 0.476099350895679, 0.46091928835187695, 0.44574189383827206, 0.43112332382010315, 0.41546724553242065, 0.4021816978310242, 0.3896732998151855, 0.3753887048717912, 0.36363059774400214, 0.35074443335526584, 0.33824610767249497, 0.32766201435288383, 0.3158918613194659, 0.3055656409731673, 0.2937381114625266, 0.28383153244319187, 0.273351947238963, 0.26330192086017323, 0.2540051974845272, 0.24436667262329562, 0.23475378381999354, 0.22519194447544197, 0.21532345853541246, 0.2070809612279943, 0.19897362957407091, 0.18949804658963235, 0.18162464841556594, 0.17352330864069246, 0.16539019955695847, 0.15718337055985224, 0.14913079901942747, -0.6474261510119071, 0.1330506780796323, 0.1258605381539013, 0.11779998963768976, 0.11122680021673763, 0.10208185688949767, 0.0965504914521418, 0.0885294144040545, 0.08116215507428624, 0.07384869969252185, 0.0671122667244253, 0.058147033019696245, 0.050876954165637735, 0.044682490723490426, 0.03828125471549274, 0.030608278071542417, 0.02241181696549984, 0.016162188587990383, 0.0087041618884185, 0.0017314088353270823, -0.007318370888902894, -0.014256168022449518, -0.02083045623792731, -0.02897436747160875, -0.037109990818159314, -0.04429750117728746, -0.05161730497008234, -0.05996180309103292, -0.06801731443805133, -0.07722715524354994, -0.08445446838480074, -0.09277539473445788, -0.10115688035700447, -0.11118007368566808, -0.12024159486268003, -0.1286570505304356, -0.1372885876419385, -0.14737913575156017, -0.15663544361171564, -0.16760601668881137, -0.17705570947669116, -0.18955684823011554, -0.20005812794822145, -0.2115047689484457, -0.2249315599132575, -0.2372867083034023, -0.2501858121674625, -0.26307542294450625, -0.27739222937148617, -0.29161106892018007, -0.308381238655305, -0.3229356517782249, -0.34152403928039826, -0.3587119729043621, -0.37684623415698965, -0.3982269963605236, -0.4185632267577112, -0.44009805730201307, -0.46452472858397004, -0.4898137030774473, -0.5154681594563403, -0.5436582913221154, -0.5753868052971625, -0.607124040065237, -0.6415641631436463, -0.6772881872440144, -0.7166782396444376, -0.7573081479172901, -0.8017270516159543, -0.8498481864407335, -0.9003524830475296, -0.9513235287518791, -1.009155593180799, -1.0669096218988718, -1.1301069542965063, -1.1950413928703931, -1.2637959112260952, -1.3304270402789815, -1.4052385614822398, -1.4776286046128246, -1.54995019837157, -1.6226413258057457, -1.694705725526286, -1.767287684058821, -1.837225393329961, -1.9022189299017398, -1.9672940303583064, -2.026961623832109, -2.085016501547923, -2.137710646154179, -2.1898199931135918, -2.237802526883711, -2.281172464441091, -2.3247171703122493, -2.3634433799077708, -2.4001809975314736, -2.436512581412944, -2.4670985970215003, -2.499386527254652, -2.5273136614812763, -2.5551413429084913, -2.580095441074831, -2.602637029174448, -2.6267391106595657, -2.6488167715503503, -2.669629795637063, -2.6875814776778753, -2.7073768546918333, -2.725283872106334, -2.742748161897122, -2.757988590230186, -2.7748996344970407, -2.7892769678451117, -2.8048643149847248, -2.8191611414300306, -2.8324616135142655, -2.844314911422705, -2.8579826539778534, -2.872089048954007, -2.884199782762025, -2.8946502816516686, -2.9078126424128174, -2.917169978723851, -2.9303080713430014, -2.941216920795811, -2.9523052455228807, -2.9616453011918993, -2.9747954498347604, -2.9835282778922783, -2.994155210789127, -3.0060391785412897, -3.016503711053161, -3.0258950223960084, -3.039292428634796, -3.0471685394120995, -3.0588628883554523, -3.0679768874598565, -3.078935883893897, -3.09142064530396, -3.1014423307741277, -3.114261077231869, -3.123306748046975, -3.1348677889942436, 3.1347626442955026, 3.1242110155276537, 3.1100276522632706, 3.098627275697003, 3.085675140947307, 3.0706070699377657, 3.0569602722840945, 3.0426705517139254, 3.027607722057268, 3.009229949151067, 2.9937351963543257, 2.976762477471132, 2.958115796112506, 2.939329888119926, 2.9190592578849324, 2.8968776899905784, 2.8749977338069113, 2.853034512187094, 2.8259014486854688, 2.8010288940819517, 2.7724006035035793, 2.7415808826640107, 2.709137304994679, 2.6752412944391457, 2.6380550884883798, 2.599045930236372, 2.5583965789942957, 2.5136831763402894, 2.466300652706757, 2.4166501247172834, 2.3634875154308466, 2.3081611208591357, 2.249240406822757, 2.187708120983702, 2.124441769391059, 2.060191792747615, 1.994278236672182, 1.9280598384360979, 1.8606037786054062, 1.7932577903878357, 1.7299405193497475, 1.666454836954993, 1.6042059874522652, 1.545623808421096, 1.4891747028762226, 1.4338353783825062, 1.38479016945561, 1.33533764413263, 1.2919628951474482, 1.2476231701500626, 1.2085161009253578, 1.1717231371959498, 1.1375952213409273, 1.107452937554854, 1.0765763575591787, 1.0490644039322188, 1.0244651507924858, 0.9976818548648808, 0.976773317322992, 0.9577413813334353, 0.9393305187309825, 0.922485277624668, 0.9029066443649627, 0.8893815018054346, 0.8719739668380028, 0.8665676757078624, 0.8494327570076123, 0.8368557053956464, 0.8294509024535597, 0.8178276549673714, 0.8109053944476666, 0.8034744997219845, 0.7962603297854153, 0.790467635324676, 0.7843524781506408, 0.777256623460905, 0.7750835887466041, 0.7736971803506136, 0.7648111148633703, 0.7658790863703647, 0.7667491253653459, 0.7640393322663126, 0.7611542091978563, 0.764696806534729, 0.7638026169535898, 0.7594577480514098, 0.7653510707902632, 0.764349048113641, 0.7688314423865208, 0.7716327791464579, 0.7724600691203451, 0.7811568037333989, 0.7828405775453979, 0.7935493561136102, 0.7985362142800956, 0.8077056449006788, 0.8157636629371818, 0.819480304047137, 0.831647964989225, 0.8401131044344927, 0.8592025690995208, 0.8699103663170566, 0.8732438019530947, 0.8938545917556884, 0.9020558954673744, 0.9146383310025706, 0.9374415017810518, 0.9519427795262136, 0.990238766001322, 0.9900154336575684, 1.0114263632438785, 1.0422271470063973, 1.065838692237985, 1.0875226094136365, 1.1144555727029584, 1.1441115295916007, 1.1659967536570823, 1.2106742892459017, 1.245521473527207, 1.2665047083019214, 1.307414245202075, 1.3485837783715906, 1.4013685192224155, 1.4312473792381444, 1.471162065318337, 1.5069397267407616, 1.5740422491794743, 1.6016692912585315, 1.6509137040461757, 1.7096839461332307, 1.758270979496239, 1.7781419107706316, 1.8464337202097976, 1.8753043403891987, 1.910320447634718, 1.9635245556276353, 1.9763424826920213, 2.033700752618906, 2.104306811637282, 2.117513018568357, 2.1417219544614943, 2.1940153828472386, 2.208787753852685, 2.229294726440969, 2.3115410362604334, 2.296949509226868, 2.329158682159559, 2.351421158935807, 2.3926944511008448, 2.397962749234472, 2.4339033584741716, 2.470929357591141, 2.430194535724556, 2.4708400768407928, 2.502135005883658, 2.5216395348357707, 2.5495914719990336, 2.5495939568975783, 2.5536917936944628, 2.5855385776781747, 2.6080659681325917, 2.6038873290907625, 2.621332901472275, 2.6322009555069075, 2.6356232322638546, 2.6531940061390844, 2.6624286883564334, 2.661148803205782, 2.6770002070526697, 2.688311937000326, 2.6840667469372117, 2.6860433548131457, 2.722835186876302, 2.7095172870959634, 2.7397636251510047, 2.720560116530783, 2.7485460115873215, 2.745135344757763, 2.7573074151186505, 2.7491978106439316, 2.7684631109546514, 2.7763152583132418, 2.7792180917438674, 2.7576445493589663, 2.7813496247984384, 2.7663095806375066, 2.7799670468102233, 2.784741202240973, 2.78440124752044, 2.7878694832013857, 2.7993808523298633, 2.7945013020962763, 2.806941529428459, 2.8096909104623813, 2.804708567305877, 2.7988160425060142, 2.811393327533493, 2.8158479261224283, 2.8290052508106664, 2.8123292505849915, 2.842392755409633, 2.8224944195413166, 2.816639263213087, 2.8452997740089008, 2.8233787578682086, 2.8170456561145873, 2.8330167216413833, 2.850302500235897, 2.841073812185231, 2.839164066720107, 2.8482583009462723, 2.838054729595992, 2.8439948957555665, 2.8367952247879535, 2.8326491375694225, 2.843644183112265, 2.859651789939188, 2.844174324901692, 2.846250138169369, 2.8437628002472164, 2.8513370792606136, 2.8399455951851245, 2.84221807667703, 2.842485925003368, 2.849306954537054, 2.8514733876954432, 2.850449655276755, 2.828042014010216, 2.832501908475115, 2.845486335056916, 2.8597600180337888, 2.8421610606132193, 2.831426174926097, 2.846065181288703, 2.8430055314226492, 2.852633419275509, 2.845718204588885, 2.8550019829387794, 2.8468620754994443, 2.8478833102509857, 2.8499866262759723, 2.841938436881183, 2.853122902802368, 2.849803769121702, 2.8470978000258444, 2.852358474258439, 2.845448740867764, 2.8627423385760626, 2.8491103584230815, 2.8323344335148004, 2.8654620545263287, 2.841013671871474, 2.848124993953119, 2.827683639295637, 2.8376622176817072, 2.829585268924845, 2.8417977120814166, 2.8260030422996847, 2.832252609974428, 2.8314424661309077, 2.8323283033423015, 2.8475625981844255, 2.8257353168766794, 2.842223639876172, 2.8393773617697105, 2.82549037222285, 2.8497489512443797, 2.801995758486477, 2.8215748190455496, 2.806586008807268, 2.816455744513318, 2.8142271213928254, 2.8064979491612543, 2.8134837438185363, 2.806288608957957, 2.799830271664184, 2.7996502507862417, 2.7991608614413326, 2.8086605313361033, 2.7993232053899932, 2.8005981957211357, 2.793560188037962, 2.7987751047425866, 2.7999748426932687, 2.795925316081786, 2.776130191488345, 2.7865990298765224, 2.7976829129556795, 2.762287302289124, 2.7854831411395864, 2.772359666859397, 2.7677361991981284, 2.7695959882758556, 2.76104594352556, 2.759177431592472, 2.775713109574355, 2.75726805003073, 2.756328302134963, 2.754752682405329, 2.753038444032271, 2.744988698873902, 2.753595713659281, 2.7325583595756435, 2.742347725481478, 2.7354307848406925, 2.7182614168907935, 2.730508666181941, 2.7220579305500223, 2.699311451327284, 2.6997994092783886, 2.7050803417923945, 2.6974301681585406, 2.700771207268545, 2.695274703615948, 2.675734338666222, 2.6779129702363464, 2.6861601143319485, 2.67823187078742, 2.656205239886389, 2.668142184443507, 2.6524151233978186, 2.656722880005459, 2.6374346247153286, 2.635563781363478, 2.6195041124213554, 2.6126551404644935, 2.6039849487468874, 2.5907554206137378, 2.5896760316484264, 2.588075764379023, 2.578800559947752, 2.566516495763698, 2.5591057206869867, 2.5436613616923025, 2.533049748492017, 2.5291313723551725, 2.5198226946709945, 2.500330811837531, 2.489970199704588, 2.471895691490707, 2.4618338778512894, 2.4656034615234073, 2.4397482295540827, 2.433922447210747, 2.408215728680277, 2.3952059212655095, 2.3775142981983985, 2.368685704598879, 2.339997409457533, 2.3231330493060183, 2.316403820998187, 2.285608390567753, 2.268448691171833, 2.2409834258912924, 2.2194642145383283, 2.1918789648034065, 2.1712997975851827, 2.1380870365360876, 2.1144235325571192, 2.0819924170799196, 2.051691697394972, 2.0263620736747177, 1.9924581446543965, 1.9517906083481424, 1.9193939859583524, 1.8810521562113183, 1.8444471797663111, 1.8087074189383912, 1.7734263234365641, 1.7297415528139477, 1.687574440345805, 1.6454530893639645, 1.5987150029758626, 1.55692438266046, 1.5162887749581415, 1.4779971727170957, 1.4237010905316954, 1.3778177965746436, 1.335015080707737, 1.2936827102374826], 10 "Freqs output":dbl[](array[numeric])=[1000.0, 1050.0, 1100.0, 1150.0, 1200.0, 1250.0, 1300.0, 1350.0, 1400.0, 1450.0, 1500.0, 1550.0, 1600.0, 1650.0, 1700.0, 1750.0, 1800.0, 1850.0, 1900.0, 1950.0, 2000.0, 2050.0, 2100.0, 2150.0, 2200.0, 2250.0, 2300.0, 2350.0, 2400.0, 2450.0, 2500.0, 2550.0, 2600.0, 2650.0, 2700.0, 2750.0, 2800.0, 2850.0, 2900.0, 2950.0, 3000.0, 3050.0, 3100.0, 3150.0, 3200.0, 3250.0, 3300.0, 3350.0, 3400.0, 3450.0, 3500.0, 3550.0, 3600.0, 3650.0, 3700.0, 3750.0, 3800.0, 3850.0, 3900.0, 3950.0, 4000.0, 4050.0, 4100.0, 4150.0, 4200.0, 4250.0, 4300.0, 4350.0, 4400.0, 4450.0, 4500.0, 4550.0, 4600.0, 4650.0, 4700.0, 4750.0, 4800.0, 4850.0, 4900.0, 4950.0, 5000.0, 5050.0, 5100.0, 5150.0, 5200.0, 5250.0, 5300.0, 5350.0, 5400.0, 5450.0, 5500.0, 5550.0, 5600.0, 5650.0, 5700.0, 5750.0, 5800.0, 5850.0, 5900.0, 5950.0, 6000.0, 6050.0, 6100.0, 6150.0, 6200.0, 6250.0, 6300.0, 6350.0, 6400.0, 6450.0, 6500.0, 6550.0, 6600.0, 6650.0, 6700.0, 6750.0, 6800.0, 6850.0, 6900.0, 6950.0, 7000.0, 7050.0, 7100.0, 7150.0, 7200.0, 7250.0, 7300.0, 7350.0, 7400.0, 7450.0, 7500.0, 7550.0, 7600.0, 7650.0, 7700.0, 7750.0, 7800.0, 7850.0, 7900.0, 7950.0, 8000.0, 8050.0, 8100.0, 8150.0, 8200.0, 8250.0, 8300.0, 8350.0, 8400.0, 8450.0, 8500.0, 8550.0, 8600.0, 8650.0, 8700.0, 8750.0, 8800.0, 8850.0, 8900.0, 8950.0, 9000.0, 9050.0, 9100.0, 9150.0, 9200.0, 9250.0, 9300.0, 9350.0, 9400.0, 9450.0, 9500.0, 9550.0, 9600.0, 9650.0, 9700.0, 9750.0, 9800.0, 9850.0, 9900.0, 9950.0, 10000.0, 10050.0, 10100.0, 10150.0, 10200.0, 10250.0, 10300.0, 10350.0, 10400.0, 10450.0, 10500.0, 10550.0, 10600.0, 10650.0, 10700.0, 10750.0, 10800.0, 10850.0, 10900.0, 10950.0, 11000.0, 11050.0, 11100.0, 11150.0, 11200.0, 11250.0, 11300.0, 11350.0, 11400.0, 11450.0, 11500.0, 11550.0, 11600.0, 11650.0, 11700.0, 11750.0, 11800.0, 11850.0, 11900.0, 11950.0, 12000.0, 12050.0, 12100.0, 12150.0, 12200.0, 12250.0, 12300.0, 12350.0, 12400.0, 12450.0, 12500.0, 12550.0, 12600.0, 12650.0, 12700.0, 12750.0, 12800.0, 12850.0, 12900.0, 12950.0, 13000.0, 13050.0, 13100.0, 13150.0, 13200.0, 13250.0, 13300.0, 13350.0, 13400.0, 13450.0, 13500.0, 13550.0, 13600.0, 13650.0, 13700.0, 13750.0, 13800.0, 13850.0, 13900.0, 13950.0, 14000.0, 14050.0, 14100.0, 14150.0, 14200.0, 14250.0, 14300.0, 14350.0, 14400.0, 14450.0, 14500.0, 14550.0, 14600.0, 14650.0, 14700.0, 14750.0, 14800.0, 14850.0, 14900.0, 14950.0, 15000.0, 15050.0, 15100.0, 15150.0, 15200.0, 15250.0, 15300.0, 15350.0, 15400.0, 15450.0, 15500.0, 15550.0, 15600.0, 15650.0, 15700.0, 15750.0, 15800.0, 15850.0, 15900.0, 15950.0, 16000.0, 16050.0, 16100.0, 16150.0, 16200.0, 16250.0, 16300.0, 16350.0, 16400.0, 16450.0, 16500.0, 16550.0, 16600.0, 16650.0, 16700.0, 16750.0, 16800.0, 16850.0, 16900.0, 16950.0, 17000.0, 17050.0, 17100.0, 17150.0, 17200.0, 17250.0, 17300.0, 17350.0, 17400.0, 17450.0, 17500.0, 17550.0, 17600.0, 17650.0, 17700.0, 17750.0, 17800.0, 17850.0, 17900.0, 17950.0, 18000.0, 18050.0, 18100.0, 18150.0, 18200.0, 18250.0, 18300.0, 18350.0, 18400.0, 18450.0, 18500.0, 18550.0, 18600.0, 18650.0, 18700.0, 18750.0, 18800.0, 18850.0, 18900.0, 18950.0, 19000.0, 19050.0, 19100.0, 19150.0, 19200.0, 19250.0, 19300.0, 19350.0, 19400.0, 19450.0, 19500.0, 19550.0, 19600.0, 19650.0, 19700.0, 19750.0, 19800.0, 19850.0, 19900.0, 19950.0, 20000.0, 20050.0, 20100.0, 20150.0, 20200.0, 20250.0, 20300.0, 20350.0, 20400.0, 20450.0, 20500.0, 20550.0, 20600.0, 20650.0, 20700.0, 20750.0, 20800.0, 20850.0, 20900.0, 20950.0, 21000.0, 21050.0, 21100.0, 21150.0, 21200.0, 21250.0, 21300.0, 21350.0, 21400.0, 21450.0, 21500.0, 21550.0, 21600.0, 21650.0, 21700.0, 21750.0, 21800.0, 21850.0, 21900.0, 21950.0, 22000.0, 22050.0, 22100.0, 22150.0, 22200.0, 22250.0, 22300.0, 22350.0, 22400.0, 22450.0, 22500.0, 22550.0, 22600.0, 22650.0, 22700.0, 22750.0, 22800.0, 22850.0, 22900.0, 22950.0, 23000.0, 23050.0, 23100.0, 23150.0, 23200.0, 23250.0, 23300.0, 23350.0, 23400.0, 23450.0, 23500.0, 23550.0, 23600.0, 23650.0, 23700.0, 23750.0, 23800.0, 23850.0, 23900.0, 23950.0, 24000.0, 24050.0, 24100.0, 24150.0, 24200.0, 24250.0, 24300.0, 24350.0, 24400.0, 24450.0, 24500.0, 24550.0, 24600.0, 24650.0, 24700.0, 24750.0, 24800.0, 24850.0, 24900.0, 24950.0, 25000.0, 25050.0, 25100.0, 25150.0, 25200.0, 25250.0, 25300.0, 25350.0, 25400.0, 25450.0, 25500.0, 25550.0, 25600.0, 25650.0, 25700.0, 25750.0, 25800.0, 25850.0, 25900.0, 25950.0, 26000.0, 26050.0, 26100.0, 26150.0, 26200.0, 26250.0, 26300.0, 26350.0, 26400.0, 26450.0, 26500.0, 26550.0, 26600.0, 26650.0, 26700.0, 26750.0, 26800.0, 26850.0, 26900.0, 26950.0, 27000.0, 27050.0, 27100.0, 27150.0, 27200.0, 27250.0, 27300.0, 27350.0, 27400.0, 27450.0, 27500.0, 27550.0, 27600.0, 27650.0, 27700.0, 27750.0, 27800.0, 27850.0, 27900.0, 27950.0, 28000.0, 28050.0, 28100.0, 28150.0, 28200.0, 28250.0, 28300.0, 28350.0, 28400.0, 28450.0, 28500.0, 28550.0, 28600.0, 28650.0, 28700.0, 28750.0, 28800.0, 28850.0, 28900.0, 28950.0, 29000.0, 29050.0, 29100.0, 29150.0, 29200.0, 29250.0, 29300.0, 29350.0, 29400.0, 29450.0, 29500.0, 29550.0, 29600.0, 29650.0, 29700.0, 29750.0, 29800.0, 29850.0, 29900.0, 29950.0, 30000.0, 30050.0, 30100.0, 30150.0, 30200.0, 30250.0, 30300.0, 30350.0, 30400.0, 30450.0, 30500.0, 30550.0, 30600.0, 30650.0, 30700.0, 30750.0, 30800.0, 30850.0, 30900.0, 30950.0, 31000.0, 31050.0, 31100.0, 31150.0, 31200.0, 31250.0, 31300.0, 31350.0, 31400.0, 31450.0, 31500.0, 31550.0, 31600.0, 31650.0, 31700.0, 31750.0, 31800.0, 31850.0, 31900.0, 31950.0, 32000.0, 32050.0, 32100.0, 32150.0, 32200.0, 32250.0, 32300.0, 32350.0, 32400.0, 32450.0, 32500.0, 32550.0, 32600.0, 32650.0, 32700.0, 32750.0, 32800.0, 32850.0, 32900.0, 32950.0, 33000.0, 33050.0, 33100.0, 33150.0, 33200.0, 33250.0, 33300.0, 33350.0, 33400.0, 33450.0, 33500.0, 33550.0, 33600.0, 33650.0, 33700.0, 33750.0, 33800.0, 33850.0, 33900.0, 33950.0, 34000.0, 34050.0, 34100.0, 34150.0, 34200.0, 34250.0, 34300.0, 34350.0, 34400.0, 34450.0, 34500.0, 34550.0, 34600.0, 34650.0, 34700.0, 34750.0, 34800.0, 34850.0, 34900.0, 34950.0, 35000.0, 35050.0, 35100.0, 35150.0, 35200.0, 35250.0, 35300.0, 35350.0, 35400.0, 35450.0, 35500.0, 35550.0, 35600.0, 35650.0, 35700.0, 35750.0, 35800.0, 35850.0, 35900.0, 35950.0, 36000.0, 36050.0, 36100.0, 36150.0, 36200.0, 36250.0, 36300.0, 36350.0, 36400.0, 36450.0, 36500.0, 36550.0, 36600.0, 36650.0, 36700.0, 36750.0, 36800.0, 36850.0, 36900.0, 36950.0, 37000.0, 37050.0, 37100.0, 37150.0, 37200.0, 37250.0, 37300.0, 37350.0, 37400.0, 37450.0, 37500.0, 37550.0, 37600.0, 37650.0, 37700.0, 37750.0, 37800.0, 37850.0, 37900.0, 37950.0, 38000.0, 38050.0, 38100.0, 38150.0, 38200.0, 38250.0, 38300.0, 38350.0, 38400.0, 38450.0, 38500.0, 38550.0, 38600.0, 38650.0, 38700.0, 38750.0, 38800.0, 38850.0, 38900.0, 38950.0, 39000.0, 39050.0, 39100.0, 39150.0, 39200.0, 39250.0, 39300.0, 39350.0, 39400.0, 39450.0, 39500.0, 39550.0, 39600.0, 39650.0, 39700.0, 39750.0, 39800.0, 39850.0, 39900.0, 39950.0, 40000.0, 40050.0, 40100.0, 40150.0, 40200.0, 40250.0, 40300.0, 40350.0, 40400.0, 40450.0, 40500.0, 40550.0, 40600.0, 40650.0, 40700.0, 40750.0, 40800.0, 40850.0, 40900.0, 40950.0, 41000.0, 41050.0, 41100.0, 41150.0, 41200.0, 41250.0, 41300.0, 41350.0, 41400.0, 41450.0, 41500.0, 41550.0, 41600.0, 41650.0, 41700.0, 41750.0, 41800.0, 41850.0, 41900.0, 41950.0, 42000.0, 42050.0, 42100.0, 42150.0, 42200.0, 42250.0, 42300.0, 42350.0, 42400.0, 42450.0, 42500.0, 42550.0, 42600.0, 42650.0, 42700.0, 42750.0, 42800.0, 42850.0, 42900.0, 42950.0, 43000.0, 43050.0, 43100.0, 43150.0, 43200.0, 43250.0, 43300.0, 43350.0, 43400.0, 43450.0, 43500.0, 43550.0, 43600.0, 43650.0, 43700.0, 43750.0, 43800.0, 43850.0, 43900.0, 43950.0, 44000.0, 44050.0, 44100.0, 44150.0, 44200.0, 44250.0, 44300.0, 44350.0, 44400.0, 44450.0, 44500.0, 44550.0, 44600.0, 44650.0, 44700.0, 44750.0, 44800.0, 44850.0, 44900.0, 44950.0, 45000.0, 45050.0, 45100.0, 45150.0, 45200.0, 45250.0, 45300.0, 45350.0, 45400.0, 45450.0, 45500.0, 45550.0, 45600.0, 45650.0, 45700.0, 45750.0, 45800.0, 45850.0, 45900.0, 45950.0, 46000.0, 46050.0, 46100.0, 46150.0, 46200.0, 46250.0, 46300.0, 46350.0, 46400.0, 46450.0, 46500.0, 46550.0, 46600.0, 46650.0, 46700.0, 46750.0, 46800.0, 46850.0, 46900.0, 46950.0, 47000.0, 47050.0, 47100.0, 47150.0, 47200.0, 47250.0, 47300.0, 47350.0, 47400.0, 47450.0, 47500.0, 47550.0, 47600.0, 47650.0, 47700.0, 47750.0, 47800.0, 47850.0, 47900.0, 47950.0, 48000.0, 48050.0, 48100.0, 48150.0, 48200.0, 48250.0, 48300.0, 48350.0, 48400.0, 48450.0, 48500.0, 48550.0, 48600.0, 48650.0, 48700.0, 48750.0, 48800.0, 48850.0, 48900.0, 48950.0, 49000.0, 49050.0, 49100.0, 49150.0, 49200.0, 49250.0, 49300.0, 49350.0, 49400.0, 49450.0, 49500.0, 49550.0, 49600.0, 49650.0, 49700.0, 49750.0, 49800.0, 49850.0, 49900.0, 49950.0, 50000.0, 50050.0, 50100.0, 50150.0, 50200.0, 50250.0, 50300.0, 50350.0, 50400.0, 50450.0, 50500.0, 50550.0, 50600.0, 50650.0, 50700.0, 50750.0, 50800.0, 50850.0, 50900.0, 50950.0, 51000.0, 51050.0, 51100.0, 51150.0, 51200.0, 51250.0, 51300.0, 51350.0, 51400.0, 51450.0, 51500.0, 51550.0, 51600.0, 51650.0, 51700.0, 51750.0, 51800.0, 51850.0, 51900.0, 51950.0, 52000.0, 52050.0, 52100.0, 52150.0, 52200.0, 52250.0, 52300.0, 52350.0, 52400.0, 52450.0, 52500.0, 52550.0, 52600.0, 52650.0, 52700.0, 52750.0, 52800.0, 52850.0, 52900.0, 52950.0, 53000.0, 53050.0, 53100.0, 53150.0, 53200.0, 53250.0, 53300.0, 53350.0, 53400.0, 53450.0, 53500.0, 53550.0, 53600.0, 53650.0, 53700.0, 53750.0, 53800.0, 53850.0, 53900.0, 53950.0, 54000.0, 54050.0, 54100.0, 54150.0, 54200.0, 54250.0, 54300.0, 54350.0, 54400.0, 54450.0, 54500.0, 54550.0, 54600.0, 54650.0, 54700.0, 54750.0, 54800.0, 54850.0, 54900.0, 54950.0, 55000.0, 55050.0, 55100.0, 55150.0, 55200.0, 55250.0, 55300.0, 55350.0, 55400.0, 55450.0, 55500.0, 55550.0, 55600.0, 55650.0, 55700.0, 55750.0, 55800.0, 55850.0, 55900.0, 55950.0, 56000.0, 56050.0, 56100.0, 56150.0, 56200.0, 56250.0, 56300.0, 56350.0, 56400.0, 56450.0, 56500.0, 56550.0, 56600.0, 56650.0, 56700.0, 56750.0, 56800.0, 56850.0, 56900.0, 56950.0, 57000.0, 57050.0, 57100.0, 57150.0, 57200.0, 57250.0, 57300.0, 57350.0, 57400.0, 57450.0, 57500.0, 57550.0, 57600.0, 57650.0, 57700.0, 57750.0, 57800.0, 57850.0, 57900.0, 57950.0, 58000.0, 58050.0, 58100.0, 58150.0, 58200.0, 58250.0, 58300.0, 58350.0, 58400.0, 58450.0, 58500.0, 58550.0, 58600.0, 58650.0, 58700.0, 58750.0, 58800.0, 58850.0, 58900.0, 58950.0, 59000.0, 59050.0, 59100.0, 59150.0, 59200.0, 59250.0, 59300.0, 59350.0, 59400.0, 59450.0, 59500.0, 59550.0, 59600.0, 59650.0, 59700.0, 59750.0, 59800.0, 59850.0, 59900.0, 59950.0, 60000.0])   [LabVIEW 2021]
doc: "Shows how to generate a standard waveform."
uses:
  <vilib>/Analysis/1siggen.llb/Ramp Pattern by Samples.vi
  <vilib>/DAQmx/read.llb/DAQmx Read (Analog 1D DBL 1Chan NSamp).vi
  <vilib>/DAQmx/write.llb/DAQmx Write (Analog Wfm 1Chan NSamp).vi
  <vilib>/DAQmx/write.llb/DAQmx Write (Analog DBL 1Chan 1Samp).vi
  <vilib>/Utility/file.llb/Read Delimited Spreadsheet (DBL).vi
  <vilib>/DAQmx/create/channels.llb/DAQmx Create Channel (AO-Voltage-Basic).vi
  <vilib>/DAQmx/configure/timing.llb/DAQmx Timing (Sample Clock).vi
  <vilib>/DAQmx/create/channels.llb/DAQmx Create Channel (AI-Voltage-Basic).vi
  <vilib>/DAQmx/configure/trigger.llb/DAQmx Start Trigger (Digital Edge).vi
  <vilib>/DAQmx/miscellaneous.llb/DAQmx Fill In Error Info.vi
  <vilib>/measure/mascope.llb/Amplitude and Levels 1 chan.vi
  <vilib>/measure/NI_MABase.lvlib
  <vilib>/Analysis/NI_AALBase.lvlib
  <vilib>/measure/NI_MAPro.lvlib
panel:
  in  "Manual Input Channels Cluster":T1={"Send amp ai-IN"="H2/ai0", "Ch2 ai -IN"="H1/ai4", "Output Chan-IN"="H2/ao0", "Ch 1 terminal config-IN"=10083, "Ch 2 terminal config-IN"=10106, "StartTrigger(use AO)-IN"="/H2/ao/StartTrigger"} {"Ch 2 terminal config-IN" items=["Default"=-1, "RSE"=10083, "NRSE"=10078, "Differential"=10106, "Pseudodifferential"=12529]; "Ch 1 terminal config-IN" items=["Default"=-1, "RSE"=10083, "NRSE"=10078, "Differential"=10106, "Pseudodifferential"=12529]}
  out "Output Chan":tag="H2/ao0"
  out "Ch 1 terminal config":i32(ring)=10083 items=["Default"=-1, "RSE"=10083, "NRSE"=10078, "Differential"=10106, "Pseudodifferential"=12529]
  out "Ch2 ai":tag="H1/ai4"
  out "Ch 2 terminal config":i32(ring)=10106 items=["Default"=-1, "RSE"=10083, "NRSE"=10078, "Differential"=10106, "Pseudodifferential"=12529]
  out "Send amp ai":tag="H2/ai0"
  out "StartTrigger(use AO)":tag="/H2/ao/StartTrigger"
  in  "Ch 2 range (max)":dbl=1.0 format="%#_13g"
  in  "Ch 1 range (max)":dbl=5.0 format="%#_13g"
  out "CH1 pk-pk":dbl=0.20894206094973328 format="%.2p"
  out "CH2 pk-pk":dbl=0.004800087986528672 format="%.2p"
  out "saved name:":string
  in  "Tab Control":T2(tab)
  out "Rogowski frequency scaling":dbl(graph)=1.0
  in  "pad time (ms)":u32=1
  in  "Freq Spacing":u16(ring) items=["Linear", "Logarithmic"]
  out "Rog Scaling":dbl=0.02412
  out "RefGain(V/A)":dbl=0.00787
  out "Techron Gain":dbl=20.0
  out "Ref_Freq":dbl=26310.0
  out "number of samples written per channel":u32
  in  "ramping samples":dbl=5000.0 format="%#_3p"
  in  "Ramping?":bool=TRUE
  out "?":cluster{"all rows":dbl[], "all rows":dbl[]}[](graph)
  in  "file (use dialog)":path=path "C:/Users/Human-MPI/Documents/GitHub/MPI_Labview_Library/Transfer Function measurement/TFRemeas_1k-500k_df50-500Hz_RxStandardProtocol.txt"
  out "Raw Inverse TF Data":dbl[][](array[numeric])
  out "Vout > Max V: set to Max V":bool
  out "Vout < 50 uV: skip":bool
  in  "MaxAllowable Vout":dbl=1.0
  in  "Save Raw Data?":bool
  in  "in:":path=path "D:/HumanImagerData"
  in  "string 2":string="TF_Tx_"
  out "freq array":dbl[](array[numeric])=[1000.0, 1050.0, 1100.0, 1150.0, 1200.0, 1250.0, 1300.0, 1350.0, 1400.0, 1450.0, 1500.0, 1550.0, 1600.0, 1650.0, 1700.0, 1750.0, 1800.0, 1850.0, 1900.0, 1950.0, 2000.0, 2050.0, 2100.0, 2150.0, 2200.0, 2250.0, 2300.0, 2350.0, 2400.0, 2450.0, 2500.0, 2550.0, 2600.0, 2650.0, 2700.0, 2750.0, 2800.0, 2850.0, 2900.0, 2950.0, 3000.0, 3050.0, 3100.0, 3150.0, 3200.0, 3250.0, 3300.0, 3350.0, 3400.0, 3450.0, 3500.0, 3550.0, 3600.0, 3650.0, 3700.0, 3750.0, 3800.0, 3850.0, 3900.0, 3950.0, 4000.0, 4050.0, 4100.0, 4150.0, 4200.0, 4250.0, 4300.0, 4350.0, 4400.0, 4450.0, 4500.0, 4550.0, 4600.0, 4650.0, 4700.0, 4750.0, 4800.0, 4850.0, 4900.0, 4950.0, 5000.0, 5050.0, 5100.0, 5150.0, 5200.0, 5250.0, 5300.0, 5350.0, 5400.0, 5450.0, 5500.0, 5550.0, 5600.0, 5650.0, 5700.0, 5750.0, 5800.0, 5850.0, 5900.0, 5950.0, 6000.0, 6050.0, 6100.0, 6150.0, 6200.0, 6250.0, 6300.0, 6350.0, 6400.0, 6450.0, 6500.0, 6550.0, 6600.0, 6650.0, 6700.0, 6750.0, 6800.0, 6850.0, 6900.0, 6950.0, 7000.0, 7050.0, 7100.0, 7150.0, 7200.0, 7250.0, 7300.0, 7350.0, 7400.0, 7450.0, 7500.0, 7550.0, 7600.0, 7650.0, 7700.0, 7750.0, 7800.0, 7850.0, 7900.0, 7950.0, 8000.0, 8050.0, 8100.0, 8150.0, 8200.0, 8250.0, 8300.0, 8350.0, 8400.0, 8450.0, 8500.0, 8550.0, 8600.0, 8650.0, 8700.0, 8750.0, 8800.0, 8850.0, 8900.0, 8950.0, 9000.0, 9050.0, 9100.0, 9150.0, 9200.0, 9250.0, 9300.0, 9350.0, 9400.0, 9450.0, 9500.0, 9550.0, 9600.0, 9650.0, 9700.0, 9750.0, 9800.0, 9850.0, 9900.0, 9950.0, 10000.0, 10050.0, 10100.0, 10150.0, 10200.0, 10250.0, 10300.0, 10350.0, 10400.0, 10450.0, 10500.0, 10550.0, 10600.0, 10650.0, 10700.0, 10750.0, 10800.0, 10850.0, 10900.0, 10950.0, 11000.0, 11050.0, 11100.0, 11150.0, 11200.0, 11250.0, 11300.0, 11350.0, 11400.0, 11450.0, 11500.0, 11550.0, 11600.0, 11650.0, 11700.0, 11750.0, 11800.0, 11850.0, 11900.0, 11950.0, 12000.0, 12050.0, 12100.0, 12150.0, 12200.0, 12250.0, 12300.0, 12350.0, 12400.0, 12450.0, 12500.0, 12550.0, 12600.0, 12650.0, 12700.0, 12750.0, 12800.0, 12850.0, 12900.0, 12950.0, 13000.0, 13050.0, 13100.0, 13150.0, 13200.0, 13250.0, 13300.0, 13350.0, 13400.0, 13450.0, 13500.0, 13550.0, 13600.0, 13650.0, 13700.0, 13750.0, 13800.0, 13850.0, 13900.0, 13950.0, 14000.0, 14050.0, 14100.0, 14150.0, 14200.0, 14250.0, 14300.0, 14350.0, 14400.0, 14450.0, 14500.0, 14550.0, 14600.0, 14650.0, 14700.0, 14750.0, 14800.0, 14850.0, 14900.0, 14950.0, 15000.0, 15050.0, 15100.0, 15150.0, 15200.0, 15250.0, 15300.0, 15350.0, 15400.0, 15450.0, 15500.0, 15550.0, 15600.0, 15650.0, 15700.0, 15750.0, 15800.0, 15850.0, 15900.0, 15950.0, 16000.0, 16050.0, 16100.0, 16150.0, 16200.0, 16250.0, 16300.0, 16350.0, 16400.0, 16450.0, 16500.0, 16550.0, 16600.0, 16650.0, 16700.0, 16750.0, 16800.0, 16850.0, 16900.0, 16950.0, 17000.0, 17050.0, 17100.0, 17150.0, 17200.0, 17250.0, 17300.0, 17350.0, 17400.0, 17450.0, 17500.0, 17550.0, 17600.0, 17650.0, 17700.0, 17750.0, 17800.0, 17850.0, 17900.0, 17950.0, 18000.0, 18050.0, 18100.0, 18150.0, 18200.0, 18250.0, 18300.0, 18350.0, 18400.0, 18450.0, 18500.0, 18550.0, 18600.0, 18650.0, 18700.0, 18750.0, 18800.0, 18850.0, 18900.0, 18950.0, 19000.0, 19050.0, 19100.0, 19150.0, 19200.0, 19250.0, 19300.0, 19350.0, 19400.0, 19450.0, 19500.0, 19550.0, 19600.0, 19650.0, 19700.0, 19750.0, 19800.0, 19850.0, 19900.0, 19950.0, 20000.0, 20050.0, 20100.0, 20150.0, 20200.0, 20250.0, 20300.0, 20350.0, 20400.0, 20450.0, 20500.0, 20550.0, 20600.0, 20650.0, 20700.0, 20750.0, 20800.0, 20850.0, 20900.0, 20950.0, 21000.0, 21050.0, 21100.0, 21150.0, 21200.0, 21250.0, 21300.0, 21350.0, 21400.0, 21450.0, 21500.0, 21550.0, 21600.0, 21650.0, 21700.0, 21750.0, 21800.0, 21850.0, 21900.0, 21950.0, 22000.0, 22050.0, 22100.0, 22150.0, 22200.0, 22250.0, 22300.0, 22350.0, 22400.0, 22450.0, 22500.0, 22550.0, 22600.0, 22650.0, 22700.0, 22750.0, 22800.0, 22850.0, 22900.0, 22950.0, 23000.0, 23050.0, 23100.0, 23150.0, 23200.0, 23250.0, 23300.0, 23350.0, 23400.0, 23450.0, 23500.0, 23550.0, 23600.0, 23650.0, 23700.0, 23750.0, 23800.0, 23850.0, 23900.0, 23950.0, 24000.0, 24050.0, 24100.0, 24150.0, 24200.0, 24250.0, 24300.0, 24350.0, 24400.0, 24450.0, 24500.0, 24550.0, 24600.0, 24650.0, 24700.0, 24750.0, 24800.0, 24850.0, 24900.0, 24950.0, 25000.0, 25050.0, 25100.0, 25150.0, 25200.0, 25250.0, 25300.0, 25350.0, 25400.0, 25450.0, 25500.0, 25550.0, 25600.0, 25650.0, 25700.0, 25750.0, 25800.0, 25850.0, 25900.0, 25950.0, 26000.0, 26050.0, 26100.0, 26150.0, 26200.0, 26250.0, 26300.0, 26350.0, 26400.0, 26450.0, 26500.0, 26550.0, 26600.0, 26650.0, 26700.0, 26750.0, 26800.0, 26850.0, 26900.0, 26950.0, 27000.0, 27050.0, 27100.0, 27150.0, 27200.0, 27250.0, 27300.0, 27350.0, 27400.0, 27450.0, 27500.0, 27550.0, 27600.0, 27650.0, 27700.0, 27750.0, 27800.0, 27850.0, 27900.0, 27950.0, 28000.0, 28050.0, 28100.0, 28150.0, 28200.0, 28250.0, 28300.0, 28350.0, 28400.0, 28450.0, 28500.0, 28550.0, 28600.0, 28650.0, 28700.0, 28750.0, 28800.0, 28850.0, 28900.0, 28950.0, 29000.0, 29050.0, 29100.0, 29150.0, 29200.0, 29250.0, 29300.0, 29350.0, 29400.0, 29450.0, 29500.0, 29550.0, 29600.0, 29650.0, 29700.0, 29750.0, 29800.0, 29850.0, 29900.0, 29950.0, 30000.0, 30050.0, 30100.0, 30150.0, 30200.0, 30250.0, 30300.0, 30350.0, 30400.0, 30450.0, 30500.0, 30550.0, 30600.0, 30650.0, 30700.0, 30750.0, 30800.0, 30850.0, 30900.0, 30950.0, 31000.0, 31050.0, 31100.0, 31150.0, 31200.0, 31250.0, 31300.0, 31350.0, 31400.0, 31450.0, 31500.0, 31550.0, 31600.0, 31650.0, 31700.0, 31750.0, 31800.0, 31850.0, 31900.0, 31950.0, 32000.0, 32050.0, 32100.0, 32150.0, 32200.0, 32250.0, 32300.0, 32350.0, 32400.0, 32450.0, 32500.0, 32550.0, 32600.0, 32650.0, 32700.0, 32750.0, 32800.0, 32850.0, 32900.0, 32950.0, 33000.0, 33050.0, 33100.0, 33150.0, 33200.0, 33250.0, 33300.0, 33350.0, 33400.0, 33450.0, 33500.0, 33550.0, 33600.0, 33650.0, 33700.0, 33750.0, 33800.0, 33850.0, 33900.0, 33950.0, 34000.0, 34050.0, 34100.0, 34150.0, 34200.0, 34250.0, 34300.0, 34350.0, 34400.0, 34450.0, 34500.0, 34550.0, 34600.0, 34650.0, 34700.0, 34750.0, 34800.0, 34850.0, 34900.0, 34950.0, 35000.0, 35050.0, 35100.0, 35150.0, 35200.0, 35250.0, 35300.0, 35350.0, 35400.0, 35450.0, 35500.0, 35550.0, 35600.0, 35650.0, 35700.0, 35750.0, 35800.0, 35850.0, 35900.0, 35950.0, 36000.0, 36050.0, 36100.0, 36150.0, 36200.0, 36250.0, 36300.0, 36350.0, 36400.0, 36450.0, 36500.0, 36550.0, 36600.0, 36650.0, 36700.0, 36750.0, 36800.0, 36850.0, 36900.0, 36950.0, 37000.0, 37050.0, 37100.0, 37150.0, 37200.0, 37250.0, 37300.0, 37350.0, 37400.0, 37450.0, 37500.0, 37550.0, 37600.0, 37650.0, 37700.0, 37750.0, 37800.0, 37850.0, 37900.0, 37950.0, 38000.0, 38050.0, 38100.0, 38150.0, 38200.0, 38250.0, 38300.0, 38350.0, 38400.0, 38450.0, 38500.0, 38550.0, 38600.0, 38650.0, 38700.0, 38750.0, 38800.0, 38850.0, 38900.0, 38950.0, 39000.0, 39050.0, 39100.0, 39150.0, 39200.0, 39250.0, 39300.0, 39350.0, 39400.0, 39450.0, 39500.0, 39550.0, 39600.0, 39650.0, 39700.0, 39750.0, 39800.0, 39850.0, 39900.0, 39950.0, 40000.0, 40050.0, 40100.0, 40150.0, 40200.0, 40250.0, 40300.0, 40350.0, 40400.0, 40450.0, 40500.0, 40550.0, 40600.0, 40650.0, 40700.0, 40750.0, 40800.0, 40850.0, 40900.0, 40950.0, 41000.0, 41050.0, 41100.0, 41150.0, 41200.0, 41250.0, 41300.0, 41350.0, 41400.0, 41450.0, 41500.0, 41550.0, 41600.0, 41650.0, 41700.0, 41750.0, 41800.0, 41850.0, 41900.0, 41950.0, 42000.0, 42050.0, 42100.0, 42150.0, 42200.0, 42250.0, 42300.0, 42350.0, 42400.0, 42450.0, 42500.0, 42550.0, 42600.0, 42650.0, 42700.0, 42750.0, 42800.0, 42850.0, 42900.0, 42950.0, 43000.0, 43050.0, 43100.0, 43150.0, 43200.0, 43250.0, 43300.0, 43350.0, 43400.0, 43450.0, 43500.0, 43550.0, 43600.0, 43650.0, 43700.0, 43750.0, 43800.0, 43850.0, 43900.0, 43950.0, 44000.0, 44050.0, 44100.0, 44150.0, 44200.0, 44250.0, 44300.0, 44350.0, 44400.0, 44450.0, 44500.0, 44550.0, 44600.0, 44650.0, 44700.0, 44750.0, 44800.0, 44850.0, 44900.0, 44950.0, 45000.0, 45050.0, 45100.0, 45150.0, 45200.0, 45250.0, 45300.0, 45350.0, 45400.0, 45450.0, 45500.0, 45550.0, 45600.0, 45650.0, 45700.0, 45750.0, 45800.0, 45850.0, 45900.0, 45950.0, 46000.0, 46050.0, 46100.0, 46150.0, 46200.0, 46250.0, 46300.0, 46350.0, 46400.0, 46450.0, 46500.0, 46550.0, 46600.0, 46650.0, 46700.0, 46750.0, 46800.0, 46850.0, 46900.0, 46950.0, 47000.0, 47050.0, 47100.0, 47150.0, 47200.0, 47250.0, 47300.0, 47350.0, 47400.0, 47450.0, 47500.0, 47550.0, 47600.0, 47650.0, 47700.0, 47750.0, 47800.0, 47850.0, 47900.0, 47950.0, 48000.0, 48050.0, 48100.0, 48150.0, 48200.0, 48250.0, 48300.0, 48350.0, 48400.0, 48450.0, 48500.0, 48550.0, 48600.0, 48650.0, 48700.0, 48750.0, 48800.0, 48850.0, 48900.0, 48950.0, 49000.0, 49050.0, 49100.0, 49150.0, 49200.0, 49250.0, 49300.0, 49350.0, 49400.0, 49450.0, 49500.0, 49550.0, 49600.0, 49650.0, 49700.0, 49750.0, 49800.0, 49850.0, 49900.0, 49950.0, 50000.0, 50050.0, 50100.0, 50150.0, 50200.0, 50250.0, 50300.0, 50350.0, 50400.0, 50450.0, 50500.0, 50550.0, 50600.0, 50650.0, 50700.0, 50750.0, 50800.0, 50850.0, 50900.0, 50950.0, 51000.0, 51050.0, 51100.0, 51150.0, 51200.0, 51250.0, 51300.0, 51350.0, 51400.0, 51450.0, 51500.0, 51550.0, 51600.0, 51650.0, 51700.0, 51750.0, 51800.0, 51850.0, 51900.0, 51950.0, 52000.0, 52050.0, 52100.0, 52150.0, 52200.0, 52250.0, 52300.0, 52350.0, 52400.0, 52450.0, 52500.0, 52550.0, 52600.0, 52650.0, 52700.0, 52750.0, 52800.0, 52850.0, 52900.0, 52950.0, 53000.0, 53050.0, 53100.0, 53150.0, 53200.0, 53250.0, 53300.0, 53350.0, 53400.0, 53450.0, 53500.0, 53550.0, 53600.0, 53650.0, 53700.0, 53750.0, 53800.0, 53850.0, 53900.0, 53950.0, 54000.0, 54050.0, 54100.0, 54150.0, 54200.0, 54250.0, 54300.0, 54350.0, 54400.0, 54450.0, 54500.0, 54550.0, 54600.0, 54650.0, 54700.0, 54750.0, 54800.0, 54850.0, 54900.0, 54950.0, 55000.0, 55050.0, 55100.0, 55150.0, 55200.0, 55250.0, 55300.0, 55350.0, 55400.0, 55450.0, 55500.0, 55550.0, 55600.0, 55650.0, 55700.0, 55750.0, 55800.0, 55850.0, 55900.0, 55950.0, 56000.0, 56050.0, 56100.0, 56150.0, 56200.0, 56250.0, 56300.0, 56350.0, 56400.0, 56450.0, 56500.0, 56550.0, 56600.0, 56650.0, 56700.0, 56750.0, 56800.0, 56850.0, 56900.0, 56950.0, 57000.0, 57050.0, 57100.0, 57150.0, 57200.0, 57250.0, 57300.0, 57350.0, 57400.0, 57450.0, 57500.0, 57550.0, 57600.0, 57650.0, 57700.0, 57750.0, 57800.0, 57850.0, 57900.0, 57950.0, 58000.0, 58050.0, 58100.0, 58150.0, 58200.0, 58250.0, 58300.0, 58350.0, 58400.0, 58450.0, 58500.0, 58550.0, 58600.0, 58650.0, 58700.0, 58750.0, 58800.0, 58850.0, 58900.0, 58950.0, 59000.0, 59050.0, 59100.0, 59150.0, 59200.0, 59250.0, 59300.0, 59350.0, 59400.0, 59450.0, 59500.0, 59550.0, 59600.0, 59650.0, 59700.0, 59750.0, 59800.0, 59850.0, 59900.0, 59950.0, 60000.0]
  out "size of saved output array":i32[](array[numeric])=[1181, 50000, 2]
  out "Output waveform (ideal)":waveform(dbl)(graph)={"t0"=timestamp(58.99999999999999 s since 1904-01-01), "dt"=1e-06, "Y"=array[50000 elements]}
  out "Output Amp":dbl=0.1
  out "CH2 Rx":dbl[](graph)
  out "CH1 Rx":dbl[](graph)
  out "delta f (Hz)":dbl
  out "stop index":i32=1180
  out "start index":i32=-1
  out "samples per channel":i32=50000
  out "ch2/ch1 phase":cluster{dbl[], dbl[]}(graph)
  out "ch2/ch1 mag":cluster{dbl[], dbl[]}(graph)
  out "current index":dbl=1180.0 format="%.2f"
  out "loop iter i":i32=1180
  out "current freq":dbl=60000.0 format="%#_6p"
  out "current Vout":dbl=0.1
  # "System Inputs"
  # "Current Channel Indicators"
  # "Note: Tx current meas and Send Amp must be on different DAQs to avoid ghosting!!"
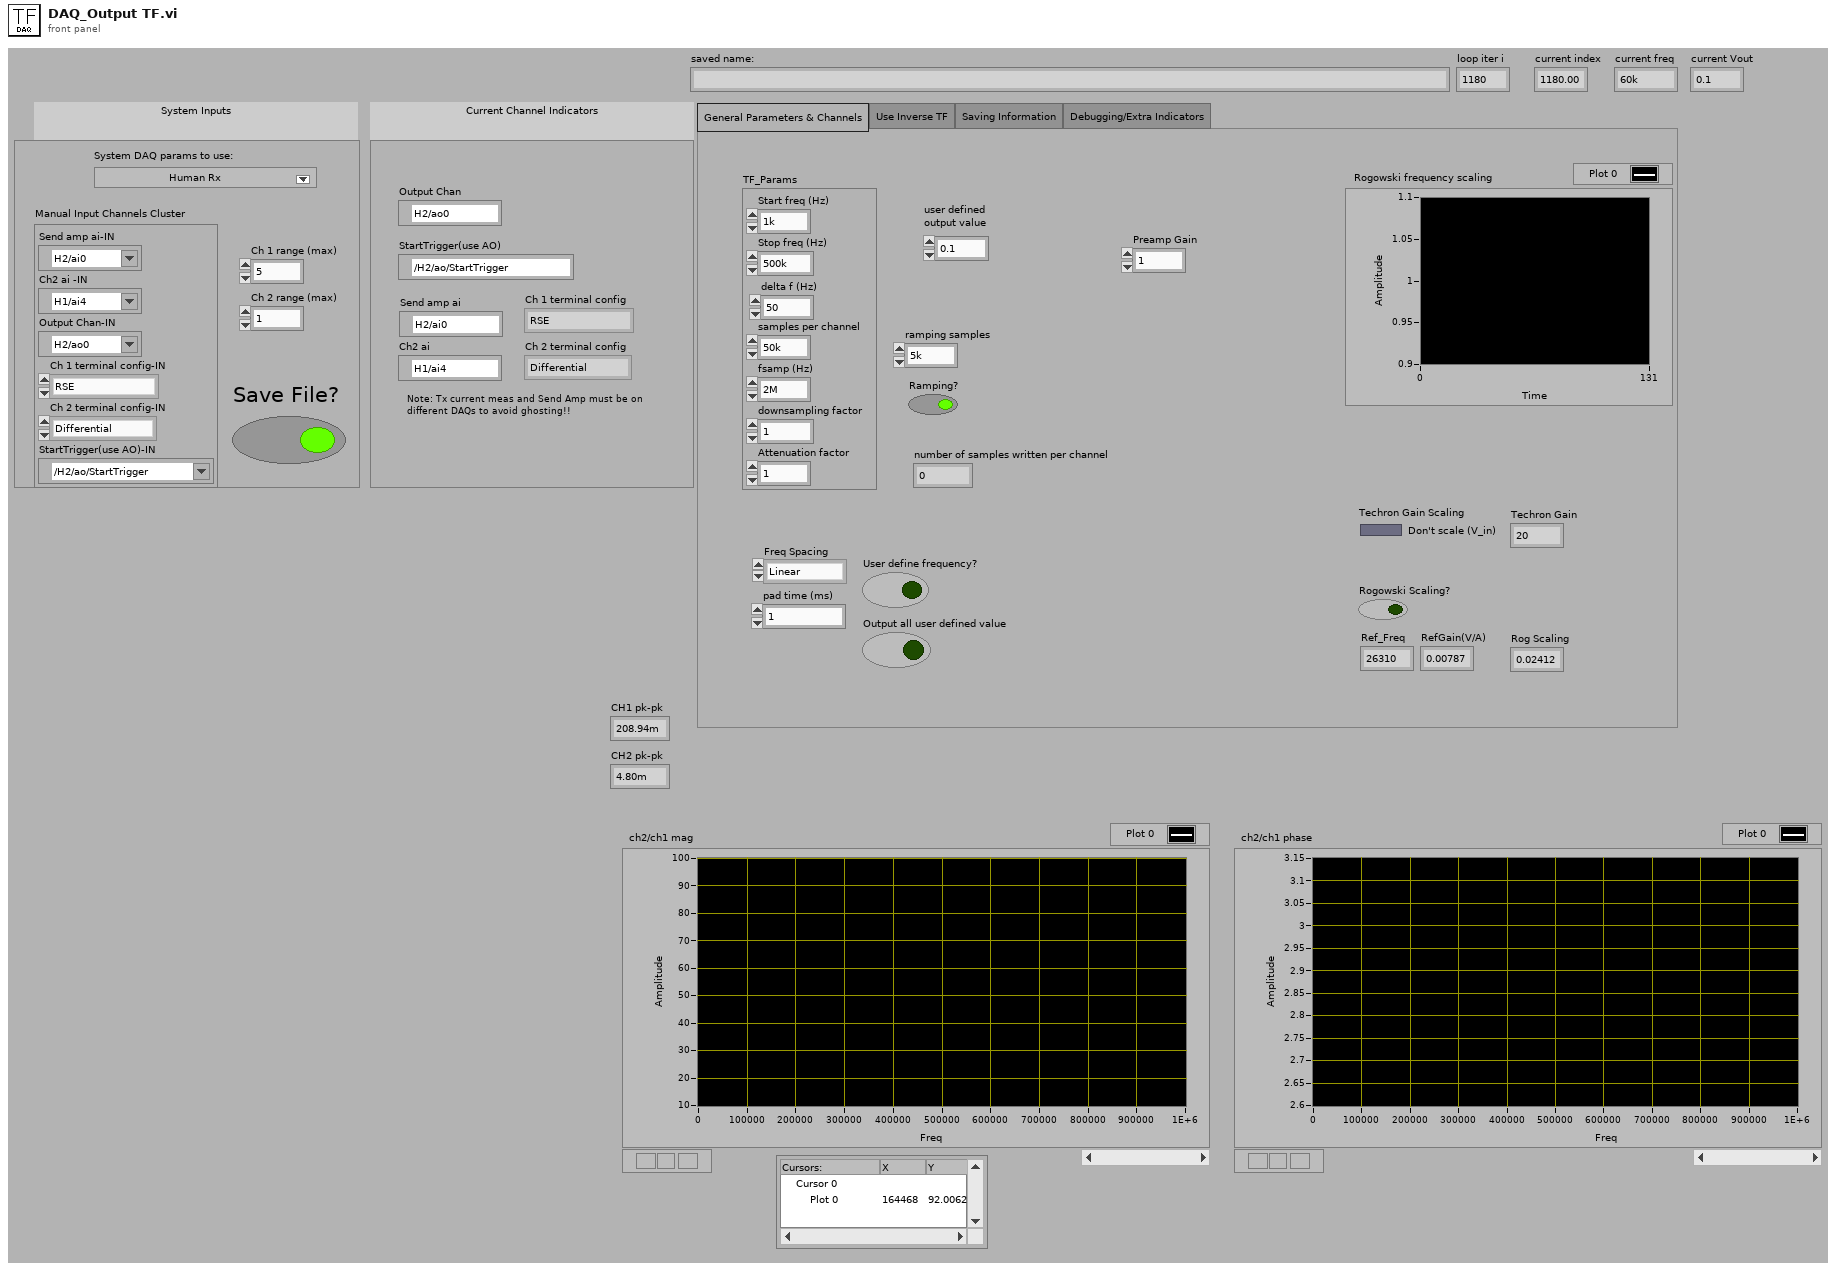
[diagram p1: front panel]
types:
  T1 = cluster{"Send amp ai-IN":tag, "Ch2 ai -IN":tag, "Output Chan-IN":tag, "Ch 1 terminal config-IN":i32, "Ch 2 terminal config-IN":i32, "StartTrigger(use AO)-IN":tag}
  T2 = enum32{"General Parameters & Channels", "Use Inverse TF", "Saving Information", "Debugging/Extra Indicators"}
  T3 = cluster{"Start freq (Hz)":dbl, "Stop freq (Hz)":dbl, "delta f (Hz)":dbl, "samples per channel":i32, "fsamp (Hz)":dbl, "downsampling factor":dbl, "Attenuation factor":dbl}
  T4 = cluster{"sample rate":dbl, "Transmit frequency":dbl, "Transmit amplitude":dbl, "sample rate digital out":dbl, "TX cycles":i32, "sample rate DAQ1":dbl, "Receive frequency":dbl, "Receive range":dbl, "TX harmonics":dbl[]}
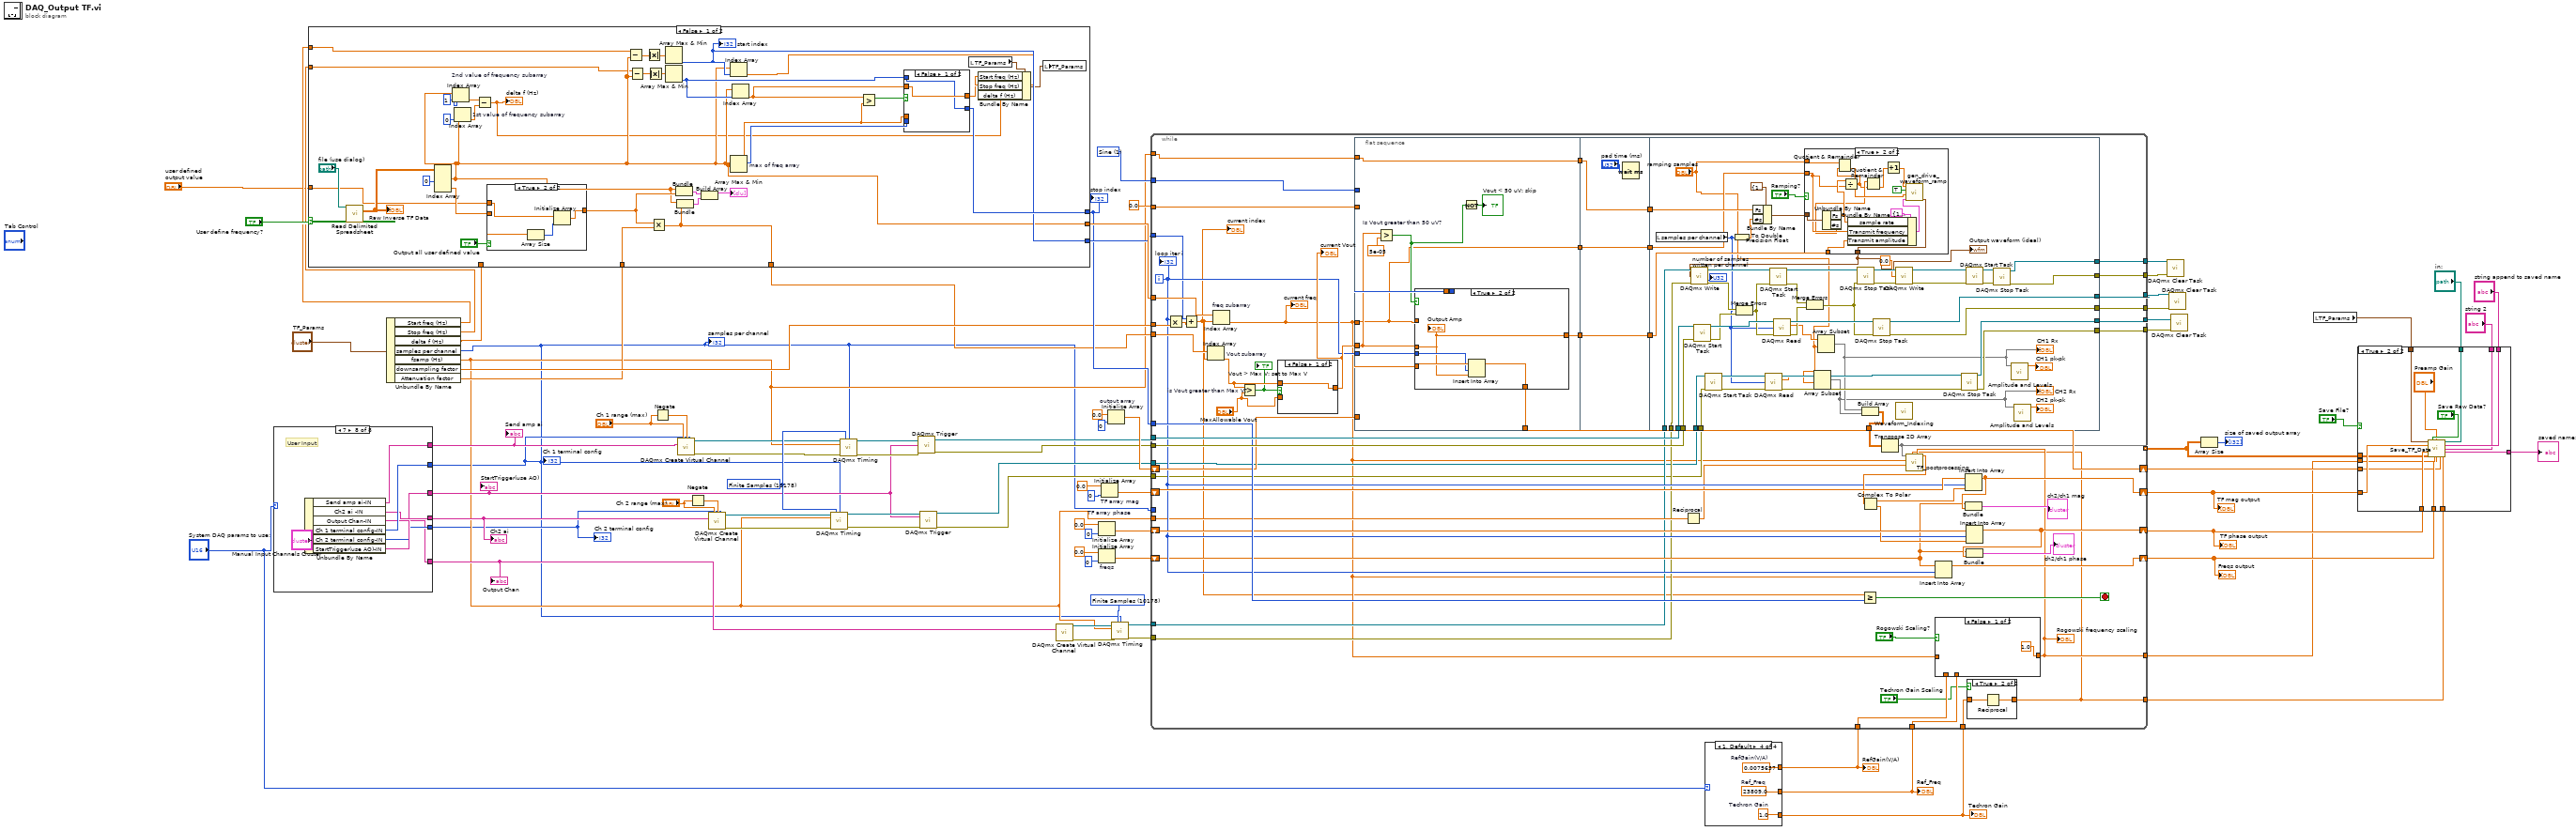
[diagram p0: block diagram]
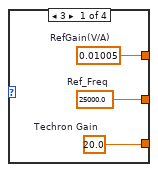
[diagram p2: hidden frame]
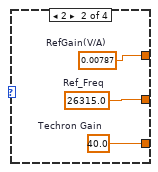
[diagram p3: hidden frame]
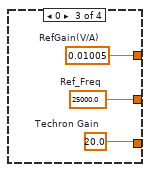
[diagram p4: hidden frame]
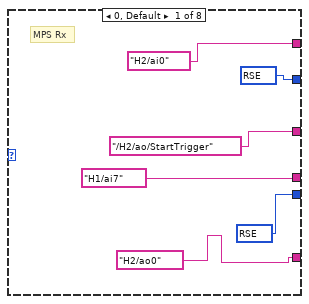
[diagram p5: hidden frame]
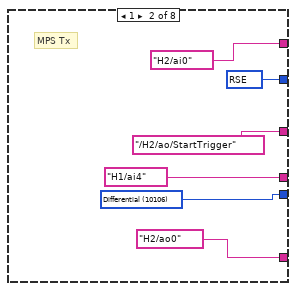
[diagram p6: hidden frame]
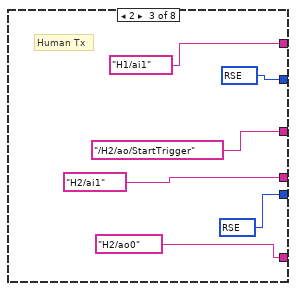
[diagram p7: hidden frame]
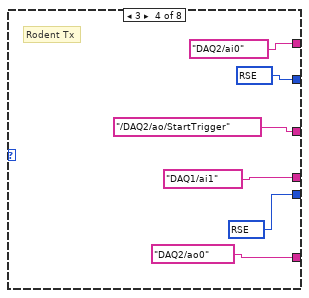
[diagram p8: hidden frame]
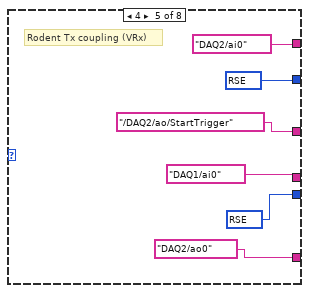
[diagram p9: hidden frame]
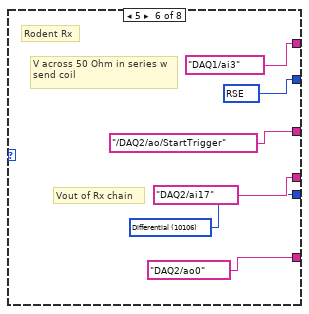
[diagram p10: hidden frame]
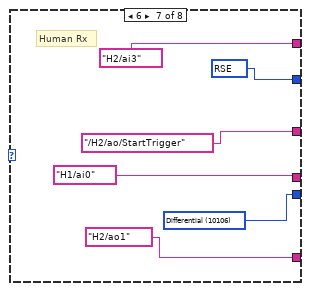
[diagram p11: hidden frame]
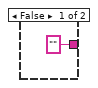
[diagram p12: hidden frame]
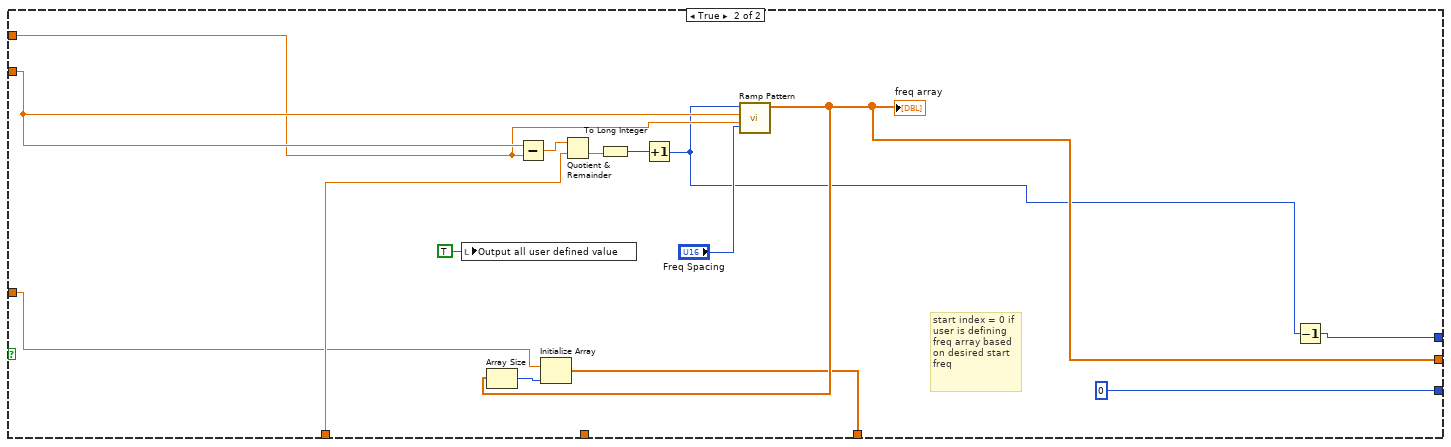
[diagram p15: hidden frame]
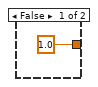
[diagram p16: hidden frame]
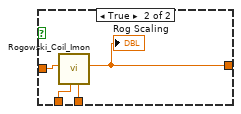
[diagram p17: hidden frame]
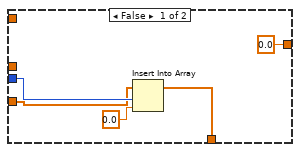
[diagram p19: hidden frame]
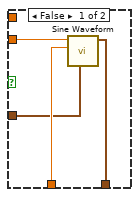
[diagram p20: hidden frame]
diagram:
  w80 = u16 1 items=["DC", "Sine", "Square", "Triangle", "Ramp", "Pulse", "Noise", "Sinc", "Negative Ramp", "Exponential Rise", "Exponential Fall", "Cardiac"] ("Waveform Function (1: Sine)")
  w55 = 10178 items=["Finite Samples"=10178, "Continuous Samples"=10123, "Hardware Timed Single Point"=12522] ("sample mode")
  w25 = 10178 items=["Finite Samples"=10178, "Continuous Samples"=10123, "Hardware Timed Single Point"=12522] ("sample mode")
  n1 = case shown="7" "System DAQ params to use:" {
    tunnel: [tag "H1/ai7" ("Tx current meas") tag "H1/ai4" ("Tx current meas") tag "H2/ai1" ("Tx current meas") tag "DAQ1/ai1" ("Tx current meas") tag "DAQ1/ai0" ("Tx current meas") tag "DAQ2/ai17" ("Tx current meas") tag "H1/ai0" ("Tx current meas") w126] -> w79
    tunnel: [tag "H2/ai0" ("Send Amp") tag "H2/ai0" ("Send Amp") tag "H1/ai1" ("Send Amp") tag "DAQ2/ai0" ("Send Amp") tag "DAQ2/ai0" ("Send Amp") tag "DAQ1/ai3" ("Send Amp") tag "H2/ai3" ("Send Amp") w127] -> w76
    tunnel: [tag "H2/ao0" ("Output Chan") tag "H2/ao0" ("Output Chan") tag "H2/ao0" ("Output Chan") tag "DAQ2/ao0" ("Output Chan") tag "DAQ2/ao0" ("Output Chan") tag "DAQ2/ao0" ("Output Chan") tag "H2/ao1" ("Output Chan") w123] -> w52
    tunnel: [tag "/H2/ao/StartTrigger" ("StartTrigger(use AO)") tag "/H2/ao/StartTrigger" ("StartTrigger(use AO)") tag "/H2/ao/StartTrigger" ("StartTrigger(use AO)") tag "/DAQ2/ao/StartTrigger" ("StartTrigger(use AO)") tag "/DAQ2/ao/StartTrigger" ("StartTrigger(use AO)") tag "/DAQ2/ao/StartTrigger" ("StartTrigger(use AO)") tag "/H2/ao/StartTrigger" ("StartTrigger(use AO)") w125] -> w24
    tunnel: [w82 w88 w94 w100 w106 w112 w119 w124] -> w3
    tunnel: [w81 w87 w93 w99 w105 w111 w121 w128] -> w2
    frame 0, Default {
      w81 = 10083 items=["Default"=-1, "RSE"=10083, "NRSE"=10078, "Differential"=10106, "Pseudodifferential"=12529] ("Ch 2 terminal config")
      w82 = 10083 items=["Default"=-1, "RSE"=10083, "NRSE"=10078, "Differential"=10106, "Pseudodifferential"=12529] ("Ch 2 terminal config")
      # "MPS Rx"
    }
    frame 1 {
      w87 = 10083 items=["Default"=-1, "RSE"=10083, "NRSE"=10078, "Differential"=10106, "Pseudodifferential"=12529] ("Ch 2 terminal config")
      w88 = 10106 items=["Default"=-1, "RSE"=10083, "NRSE"=10078, "Differential"=10106, "Pseudodifferential"=12529] ("Ch 2 terminal config")
      # "MPS Tx"
    }
    frame 2 {
      w93 = 10083 items=["Default"=-1, "RSE"=10083, "NRSE"=10078, "Differential"=10106, "Pseudodifferential"=12529] ("Ch 2 terminal config")
      w94 = 10083 items=["Default"=-1, "RSE"=10083, "NRSE"=10078, "Differential"=10106, "Pseudodifferential"=12529] ("Ch 2 terminal config")
      # "Human Tx"
    }
    frame 3 {
      w99 = 10083 items=["Default"=-1, "RSE"=10083, "NRSE"=10078, "Differential"=10106, "Pseudodifferential"=12529] ("Ch 2 terminal config")
      w100 = 10083 items=["Default"=-1, "RSE"=10083, "NRSE"=10078, "Differential"=10106, "Pseudodifferential"=12529] ("Ch 2 terminal config")
      # "Rodent Tx"
    }
    frame 4 {
      w105 = 10083 items=["Default"=-1, "RSE"=10083, "NRSE"=10078, "Differential"=10106, "Pseudodifferential"=12529] ("Ch 2 terminal config")
      w106 = 10083 items=["Default"=-1, "RSE"=10083, "NRSE"=10078, "Differential"=10106, "Pseudodifferential"=12529] ("Ch 2 terminal config")
      # "Rodent Tx coupling (VRx)"
    }
    frame 5 {
      w111 = 10083 items=["Default"=-1, "RSE"=10083, "NRSE"=10078, "Differential"=10106, "Pseudodifferential"=12529] ("Ch 2 terminal config")
      w112 = 10106 items=["Default"=-1, "RSE"=10083, "NRSE"=10078, "Differential"=10106, "Pseudodifferential"=12529] ("Ch 2 terminal config")
      # "V across 50 Ohm in series w send coil"
      # "Vout of Rx chain"
      # "Rodent Rx"
    }
    frame 6 {
      w121 = 10083 items=["Default"=-1, "RSE"=10083, "NRSE"=10078, "Differential"=10106, "Pseudodifferential"=12529] ("Ch 2 terminal config")
      w119 = 10106 items=["Default"=-1, "RSE"=10083, "NRSE"=10078, "Differential"=10106, "Pseudodifferential"=12529] ("Ch 2 terminal config")
      # "Human Rx"
    }
    frame 7 {
      # "User Input"
      n2 = Unbundle By Name("Manual Input Channels Cluster") -> ("Send amp ai-IN"=w127:tag, "Ch2 ai -IN"=w126:tag, "Output Chan-IN"=w123:tag, "Ch 1 terminal config-IN"=w128:i32, "Ch 2 terminal config-IN"=w124:i32, "StartTrigger(use AO)-IN"=w125:tag)
    }
  }
  "Ch 2 terminal config" <- w3
  "Ch 1 terminal config" <- w2
  "Output Chan" <- w52
  "Ch2 ai" <- w79
  "StartTrigger(use AO)" <- w24
  "Send amp ai" <- w76
  n3 = Unbundle By Name("TF_Params") -> ("Start freq (Hz)"=w36:dbl, "Stop freq (Hz)"=w35:dbl, "delta f (Hz)"=w34:dbl, "samples per channel"=w1:i32, "fsamp (Hz)"=w8:dbl, "downsampling factor"=w38:dbl, "Attenuation factor"=w37:dbl)
  "samples per channel" <- w1
  n4 = case shown="False" "User define frequency?" {
    tunnel: [w140 w179] -> w48
    tunnel: [w141 0] -> w47
    tunnel: [w142 w175] -> w46
    tunnel: w37 -> [w139 _]
    tunnel: w36 -> [w134 w183]
    tunnel: w35 -> [w133 w184]
    tunnel: w34 -> [_ w185]
    tunnel: "user defined \noutput value" -> [w131 w178]
    tunnel: [w130 w177] -> w28
    frame False {
      n5 = call-poly <vilib>:"Read Delimited Spreadsheet.vi"("file path (dialog if empty)"="file (use dialog)") -> ("all rows"=w149:dbl[][])  [unwired: 9 in, 5 out]
      "Raw Inverse TF Data" <- w149
      n6 = Index Array(array=w149, index (col) #1=0 ("disabled index (col)")) -> (element #1=w140:dbl[], element #2=w162:dbl[])  [unwired: 3 in]
      n7 = Index Array "2nd value of frequency subarray"(array=w140, index=1) -> (element=w148:dbl)
      n8 = Index Array "1st value of frequency subarray"(array=w140, index=0) -> (element=w147:dbl)
      n9 = Subtract(x=w148, y=w147) -> (x-y=w132:dbl)
      "delta f (Hz)" <- w132
      n10 = case shown="True" "Output all user defined value" {
        tunnel: w162 -> [w165 w169]
        tunnel: [w165 w167] -> w164
        tunnel: w131 -> [_ w166]
        frame False {
        }
        frame True {
          n11 = Array Size(array=w169) -> (size(s)=w168:i32)
          n12 = Initialize Array(w166, w168) -> (w167:dbl[])
        }
      }
      n13 = Subtract(x=w134, y=w140) -> (x-y=w150:dbl[])
      n14 = Subtract(x=w133, y=w140) -> (x-y=w152:dbl[])
      n15 = Absolute Value(x=w150) -> (abs(x)=w151:dbl[])
      n16 = Absolute Value(x=w152) -> (abs(x)=w153:dbl[])
      n17 = Multiply(x=w164, y=w139) -> (x*y=w130:dbl[])
      n18 = Array Max & Min(array=w151) -> (min index (indices)=w141:i32)  [unwired: 3 out]
      "start index" <- w141
      n19 = Array Max & Min(array=w153) -> (min index (indices)=w157:i32)  [unwired: 3 out]
      n20 = Bundle("all rows"=w140, "all rows"=w164) -> (w160:cluster{"all rows":dbl[], "all rows":dbl[]})  [unwired: 1 in]
      n21 = Bundle("all rows"=w140, w130) -> (w159:cluster{"all rows":dbl[], dbl[]})  [unwired: 1 in]
      n22 = Build Array(w160, w159) -> (→"?":cluster{"all rows":dbl[], "all rows":dbl[]}[])
      n23 = Index Array(array=w140, index=w141) -> (element=w136:dbl)
      n24 = Array Max & Min "max of freq array"(array=w140) -> (max value=w156:dbl, max index (indices)=w158:i32)  [unwired: 2 out]
      n25 = Index Array(array=w140, index=w157) -> (element=w155:dbl)
      n26 = Greater?(x=w155, y=w156) -> (0:w154:bool)
      n27 = case shown="False" w154 {
        tunnel: [w171 w173] -> w135
        tunnel: w156 -> [_ w173]
        tunnel: w155 -> [w171 _]
        tunnel: w157 -> [w170 _]
        tunnel: w158 -> [_ w172]
        tunnel: [w170 w172] -> w142
        frame False {
        }
        frame True {
        }
      }
      n28 = local read "TF_Params"() -> (w138:T3)
      n29 = Bundle By Name(cluster=w138, "Start freq (Hz)"=w136, "Stop freq (Hz)"=w135, "delta f (Hz)"=w132) -> (w137:T3)
      n30 = local write "TF_Params"(w137) -> ()
    }
    frame True {
      # "start index = 0 if user is defining freq array based\non desired start freq"
      n31 = local write "Output all user defined value"(TRUE ("Output all user defined value")) -> ()
      n32 = Subtract(x=w184, y=w183) -> (x-y=w186:dbl)
      n33 = Quotient & Remainder(x=w186, y=w185) -> (floor(x/y)=w187:dbl)  [unwired: 1 out]
      n34 = To Long Integer(number=w187) -> (32bit integer=w176:i32)
      n35 = Increment(x=w176) -> (x+1=w174:i32)
      n36 = call-poly <vilib>:"Ramp Pattern.vi"("type"="Freq Spacing", "start"=w183, "end"=w184, "samples"=w174) -> ("Ramp Pattern"=w179:dbl[])  [unwired: 6 in, 1 out]
      "freq array" <- w179
      n37 = Array Size(array=w179) -> (size(s)=w180:i32)
      n38 = Initialize Array(w178, w180) -> (w177:dbl[])
      n39 = Decrement(x=w174) -> (x-1=w175:i32)
    }
  }
  "stop index" <- w46
  n40 = Negate(x="Ch 1 range (max)") -> (-x=w4:dbl)
  n41 = call-poly <vilib>:"DAQmx Create Virtual Channel.vi"("maximum value"="Ch 1 range (max)", "minimum value"=w4, "input terminal configuration"=w2, "physical channels"=w76) -> ("task out"=w21:refnum<k21>, "error out"=w20:errorcluster)  [unwired: 10 in]
  n42 = Negate(x="Ch 2 range (max)") -> (-x=w7:dbl)
  n43 = call-poly <vilib>:"DAQmx Create Virtual Channel.vi"("maximum value"="Ch 2 range (max)", "minimum value"=w7, "input terminal configuration"=w3, "physical channels"=w79) -> ("task out"=w22:refnum<k21>, "error out"=w23:errorcluster)  [unwired: 10 in]
  n44 = call-poly <vilib>:"DAQmx Timing.vi"("task/channels in"=w22, "sample mode"=w25, "samples per channel"=w1, "rate"=w8, "error in"=w23) -> ("task out"=w27:refnum<k21>, "error out"=w26:errorcluster)  [unwired: 9 in]
  n45 = call-poly <vilib>:"DAQmx Timing.vi"("task/channels in"=w21, "sample mode"=w25, "samples per channel"=w1, "rate"=w8, "error in"=w20) -> ("task out"=w61:refnum<k21>, "error out"=w58:errorcluster)  [unwired: 9 in]
  n46 = call-poly <vilib>:"DAQmx Trigger.vi"("task/channels in"=w61, "source"=w24, "error in"=w58) -> ("task out"=w60:refnum<k21>, "error out"=w59:errorcluster)  [unwired: 11 in]
  n47 = call-poly <vilib>:"DAQmx Trigger.vi"("task/channels in"=w27, "source"=w24, "error in"=w26) -> ("task out"=w16:refnum<k21>, "error out"=w19:errorcluster)  [unwired: 11 in]
  n48 = call-poly <vilib>:"DAQmx Create Virtual Channel.vi"("physical channels"=w52) -> ("task out"=w57:refnum<k21>, "error out"=w56:errorcluster)  [unwired: 13 in]
  n49 = Initialize Array "freqs"(0.0 ("element"), 0 ("dimension size")) -> (w62:dbl[])
  n50 = Initialize Array "TF array phase"(0.0 ("element"), 0 ("dimension size")) -> (w65:dbl[])
  n51 = Initialize Array "TF array mag"(0.0 ("element"), 0 ("dimension size")) -> (w68:dbl[])
  n52 = Initialize Array "output array"(0.0 ("element"), 0 ("dimension size")) -> (w71:dbl[])
  n53 = call-poly <vilib>:"DAQmx Timing.vi"("task/channels in"=w57, "sample mode"=w55, "samples per channel"=w1, "rate"=w8, "error in"=w56) -> ("task out"=w54:refnum<k21>, "error out"=w53:errorcluster)  [unwired: 9 in]
  n54 = case shown="1, Default" "System DAQ params to use:" {
    tunnel: [w189 w194 w195 w200] -> w12
    tunnel: [w190 w193 w196 w199] -> w11
    tunnel: [w191 w192 w197 w198] -> w10
    frame 3 {
      w190 = 25000.0  # Ref_Freq
      w189 = 0.01005  # RefGain(V/A)
      w191 = 20.0  # Techron Gain
    }
    frame 2 {
      w193 = 26315.0  # Ref_Freq
      w194 = 0.00787  # RefGain(V/A)
      w192 = 40.0  # Techron Gain
    }
    frame 0 {
      w196 = 25000.0  # Ref_Freq
      w195 = 0.01005  # RefGain(V/A)
      w197 = 20.0  # Techron Gain
    }
    frame 1, Default {
      w199 = 23809.0  # Ref_Freq
      w200 = 0.0075657  # RefGain(V/A)
      w198 = 1.0  # Techron Gain
    }
  }
  "Techron Gain" <- w10
  "Ref_Freq" <- w11
  "RefGain(V/A)" <- w12
  n55 = while {
    tunnel: w80 -> [w259]
    tunnel: [w241] -> w40 mode=indexing
    tunnel: w28 -> [w253]
    tunnel: w48 -> [w236]
    tunnel: w38 -> [w252]
    tunnel: 0.0 ("DC Offset (0.00 V)") -> [w248]
    tunnel: w46 -> [w247]
    shift-right: [w243] -> w39
    shift-left: w71 -> [w244]
    tunnel: w1 -> [_]
    tunnel: w8 -> [w226]
    shift-right: [w232] -> w42
    shift-left: w68 -> [w240]
    shift-right: [w230] -> w41
    shift-left: w65 -> [w239]
    shift-right: [w234] -> w43
    shift-left: w62 -> [w229]
    tunnel: w54 -> [w225]
    tunnel: w53 -> [w224]
    tunnel: [w219] -> w50
    tunnel: [w218] -> w51
    tunnel: w47 -> [w217]
    tunnel: w19 -> [w216]
    tunnel: [w215] -> w18
    tunnel: [w214] -> w17
    tunnel: w16 -> [w213]
    tunnel: w60 -> [w258]
    tunnel: [w256] -> w78
    tunnel: w59 -> [w257]
    tunnel: [w254] -> w77
    tunnel: [w205] -> w14
    tunnel: [w210] -> w13
    tunnel: w12 -> [w209]
    tunnel: w11 -> [w208]
    tunnel: w10 -> [w206]
    tunnel: w8 -> [w204]
    i -> [w235]
    stop <- w246 stop-if-true
    n56 = Multiply(x=w235, y=w252) -> (x*y=w245:dbl)
    n57 = Add(x=w217, y=w245) -> (x+y=w201:dbl)
    "current index" <- w201
    n58 = Index Array "Vout subarray"(array=w253, index=w201) -> (element=w251:dbl)
    n59 = Index Array "freq subarray"(array=w236, index=w201) -> (element=w211:dbl)
    "current freq" <- w211
    n60 = Greater? "is Vout greater than Max V?"(x=w251, y="MaxAllowable Vout") -> (0:w249:bool)
    "Vout > Max V: set to Max V" <- w249
    n61 = case shown="False" w249 {
      tunnel: [w268 w269] -> w250
      tunnel: "MaxAllowable Vout" -> [_ w269]
      tunnel: w251 -> [w268 _]
      frame False {
      }
      frame True {
      }
    }
    "current Vout" <- w250
    n62 = flat-sequence {
      tunnel: w250 -> [w279]
      tunnel: w259 -> [w281]
      tunnel: w211 -> [w272]
      tunnel: w248 -> [w280]
      tunnel: w244 -> [w275]
      tunnel: w235 -> [w274]
      tunnel: [w273] -> w243
      tunnel: [w272] -> w223
      tunnel: [w271] -> w221
      tunnel: w204 -> [w270]
      tunnel: [w270] -> w203
      tunnel: w223 -> [w293]
      tunnel: [w293] -> w222
      tunnel: w221 -> [w292]
      tunnel: [w292] -> w220
      tunnel: w203 -> [w291]
      tunnel: [w291] -> w202
      tunnel: w258 -> [w344]
      tunnel: w257 -> [w341]
      tunnel: [w342] -> w256
      tunnel: [w310] -> w255
      tunnel: [w332] -> w254
      tunnel: w225 -> [w340]
      tunnel: w224 -> [w339]
      tunnel: w222 -> [w301]
      tunnel: w220 -> [w338]
      tunnel: [w321] -> w219
      tunnel: [w320] -> w218
      tunnel: w216 -> [w318]
      tunnel: [w316] -> w215
      tunnel: [w315] -> w214
      tunnel: w213 -> [w312]
      tunnel: w202 -> [w304]
      frame #0 {
        n63 = Greater? "Is Vout greater than 50 uV?"(x=w279, y=5e-05) -> (0:w277:bool)
        n64 = case shown="True" w277 {
          tunnel: w279 -> [_ w287]
          tunnel: w281 -> [_ _]
          tunnel: w272 -> [_ _]
          tunnel: w280 -> [_ _]
          tunnel: w275 -> [w285 w290]
          tunnel: w274 -> [w286 w289]
          tunnel: [w283 w288] -> w273
          tunnel: [0.0 ("y") w287] -> w271
          frame False {
            n65 = Insert Into Array(array=w285, index=w286, new element=0.0 ("new element/subarray")) -> (w283:dbl[])
          }
          frame True {
            n66 = Insert Into Array(array=w290, index=w289, new element=w287) -> (w288:dbl[])
            "Output Amp" <- w287
          }
        }
        n67 = Not(x=w277) -> (.not. x?=→"Vout < 50 uV: skip":bool)
      }
      frame #1 {
        n68 = Wait (ms)(milliseconds to wait="pad time (ms)") -> ()  [unwired: 1 out]
      }
      frame #2 {
        n69 = local read "samples per channel"() -> (w311:i32)
        n70 = call <vilib>:"DAQmx Start Task.vi"("task/channels in"=w344, "error in"=w341) -> ("task out"=w345:refnum<k21>, "error out"=w337:errorcluster)  [unwired: 12 in]
        n71 = call <vilib>:"DAQmx Start Task.vi"("task/channels in"=w312, "error in"=w318) -> ("task out"=w313:refnum<k21>, "error out"=w308:errorcluster)  [unwired: 12 in]
        n72 = To Double Precision Float(number=w311) -> (double precision float=w330:dbl)
        n73 = Bundle By Name(cluster=cluster{"Fs":dbl, "#s":dbl} {"Fs"=1000.0, "#s"=1000.0} ("sampling info"), "Fs"=w304, "#s"=w330) -> (w329:cluster{"Fs":dbl, "#s":dbl})
        n74 = call-poly <vilib>:"DAQmx Read.vi"("task/channels in"=w313, "number of samples per channel"=w311, "error in"=w308) -> ("task out"=w314:refnum<k21>, "data"=w299:dbl[], "error out"=w307:errorcluster)  [unwired: 10 in]
        n75 = case shown="True" "Ramping?" {
          tunnel: w301 -> [w349 w353]
          tunnel: w338 -> [w348 w361]
          tunnel: w329 -> [w347 w362]
          tunnel: [w346 w358] -> w297
          tunnel: "ramping samples" -> [_ w357]
          frame False {
            n76 = call <vilib>:"Sine Waveform.vi"("sampling info"=w347, "amplitude"=w348, "frequency"=w349) -> ("signal out"=w346:waveform(dbl))  [unwired: 7 in, 1 out]
          }
          frame True {
            n77 = Unbundle By Name(w362) -> ("Fs"=w354:dbl, "#s"=w352:dbl)
            n78 = Divide(x=w354, y=w353) -> (x/y=w350:dbl)
            n79 = Quotient & Remainder(x=w357, y=w350) -> (floor(x/y)=w356:dbl)  [unwired: 1 out]
            n80 = Bundle By Name(cluster=T4 {"sample rate"=1000000.0, "Transmit frequency"=25000.0, "Transmit amplitude"=1.577, "sample rate digital out"=40000.0, "TX cycles"=600, "sample rate DAQ1"=1000000.0, "Receive frequency"=75000.0, "Receive range"=1.0, "TX harmonics"=[50000.0, 75000.0, 100000.0, 125000.0, 150000.0, 175000.0, 200000.0, 225000.0]} ("TxRxParams"), "sample rate"=w354, "Transmit frequency"=w353, "Transmit amplitude"=w361) -> (w359:T4)
            n81 = Quotient & Remainder(x=w352, y=w350) -> (floor(x/y)=w351:dbl)  [unwired: 1 out]
            n82 = Increment(x=w351) -> (x+1=w355:dbl)
            n83 = call "gen_drive_waveform_ramp.vi"("TxRxParams"=w359, "ramping cycles"=w356, "ramping?"=TRUE, "no of cycles"=w355) -> ("signal out"=w358:waveform(dbl))  [unwired: 7 in]
          }
        }
        "Output waveform (ideal)" <- w297
        n84 = call-poly <vilib>:"DAQmx Write.vi"("task/channels in"=w340, "data"=w297, "error in"=w339) -> ("task out"=w335:refnum<k21>, "number of samples written per channel"=→"number of samples written per channel":u32, "error out"=w336:errorcluster)  [unwired: 10 in]
        n85 = Merge Errors(w336, w337) -> (w317:errorcluster)
        n86 = call <vilib>:"DAQmx Start Task.vi"("task/channels in"=w335, "error in"=w317) -> ("task out"=w331:refnum<k21>, "error out"=w333:errorcluster)  [unwired: 12 in]
        n87 = call-poly <vilib>:"DAQmx Read.vi"("task/channels in"=w345, "number of samples per channel"=w311, "error in"=w317) -> ("task out"=w343:refnum<k21>, "data"=w303:dbl[], "error out"=w334:errorcluster)  [unwired: 10 in]
        n88 = Merge Errors(w333, w334) -> (w309:errorcluster)
        n89 = Array Subset(array=w299, index="ramping samples") -> (w300:dbl[])  [unwired: 1 in]
        "CH2 Rx" <- w300
        n90 = Array Subset(array=w303, index="ramping samples") -> (w302:dbl[])  [unwired: 1 in]
        "CH1 Rx" <- w302
        n91 = call <vilib>:"DAQmx Stop Task.vi"("task/channels in"=w331, "error in"=w309) -> ("task out"=w325:refnum<k21>, "error out"=w324:errorcluster)  [unwired: 12 in]
        n92 = Build Array(w302, w300) -> (w310:dbl[][])
        n93 = call <vilib>:"DAQmx Stop Task.vi"("task/channels in"=w343, "error in"=w309) -> ("task out"=w342:refnum<k21>, "error out"=w332:errorcluster)  [unwired: 12 in]
        n94 = call-poly <vilib>:"DAQmx Write.vi"("task/channels in"=w325, "data"=0.0, "error in"=w324) -> ("task out"=w326:refnum<k21>, "error out"=w327:errorcluster)  [unwired: 10 in, 1 out]
        n95 = call "Waveform_Indexing.vi"() -> ()  [unwired: 9 in, 1 out]
        n96 = call <vilib>:"DAQmx Stop Task.vi"("task/channels in"=w314, "error in"=w307) -> ("task out"=w315:refnum<k21>, "error out"=w316:errorcluster)  [unwired: 12 in]
        n97 = call <vilib>:"DAQmx Start Task.vi"("task/channels in"=w326, "error in"=w327) -> ("task out"=w323:refnum<k21>, "error out"=w322:errorcluster)  [unwired: 12 in]
        n98 = call <vilib>:"DAQmx Stop Task.vi"("task/channels in"=w323, "error in"=w322) -> ("task out"=w321:refnum<k21>, "error out"=w320:errorcluster)  [unwired: 12 in]
        n99 = call-poly <vilib>:"Amplitude and Levels.vi"("signal in"=w302) -> ("amplitude"=→"CH1 pk-pk":dbl)  [unwired: 7 in, 3 out]
        n100 = call-poly <vilib>:"Amplitude and Levels.vi"("signal in"=w300) -> ("amplitude"=→"CH2 pk-pk":dbl)  [unwired: 7 in, 3 out]
      }
    }
    n101 = Reciprocal(x=w226) -> (1/x=w227:dbl)
    n102 = Greater Or Equal?(x=w201, y=w247) -> (x >= y?=w246:bool)
    n103 = Transpose 2D Array(2D array=w255) -> (transposed array=w241:dbl[][])
    n104 = Insert Into Array(array=w229, index=w235, new element=w211) -> (w234:dbl[])
    n105 = case shown="False" "Rogowski Scaling?" {
      tunnel: w211 -> [_ w267]
      tunnel: [1.0 ("x*y") w266] -> w210
      tunnel: w209 -> [_ w265]
      tunnel: w208 -> [_ w264]
      frame False {
      }
      frame True {
        n106 = call "Rogowski_Coil_Imon.vi"("Ref_Freq"=w264, "RefGain"=w265, "CurrentFreq"=w267) -> ("x*y"=w266:dbl)  [unwired: 8 in]
        "Rog Scaling" <- w266
      }
    }
    "Rogowski frequency scaling" <- w210
    n107 = case shown="True" "Techron Gain Scaling" {
      tunnel: w206 -> [_ w262]
      tunnel: [1.0 w261] -> w205
      frame False {
      }
      frame True {
        n108 = Reciprocal(x=w262) -> (1/x=w261:dbl)
      }
    }
    n109 = call "TF_postprocessing.vi"("Div ch2 by:"=w210, "Div ch1 by:"=w205, "dt"=w227, "current frequency"=w211, "data"=w241) -> ("ch2/ch1"=w238:cdb)  [unwired: 6 in]
    n110 = Complex To Polar(r * e^(i*theta)=w238) -> (r=w233:dbl, theta=w237:dbl)
    n111 = Insert Into Array(array=w240, index=w235, new element=w233) -> (w232:dbl[])
    n112 = Bundle(w229, w232) -> (→"ch2/ch1 mag":cluster{dbl[], dbl[]})  [unwired: 1 in]
    n113 = Insert Into Array(array=w239, index=w235, new element=w237) -> (w230:dbl[])
    n114 = Bundle(w229, w230) -> (→"ch2/ch1 phase":cluster{dbl[], dbl[]})  [unwired: 1 in]
    "loop iter i" <- w235
  }
  "Freqs output" <- w43
  "TF mag output" <- w42
  "TF phase output" <- w41
  n115 = call <vilib>:"DAQmx Clear Task.vi"("task in"=w50, "error in"=w51) -> ()  [unwired: 13 in, 1 out]
  n116 = call <vilib>:"DAQmx Clear Task.vi"("task in"=w78, "error in"=w77) -> ()  [unwired: 13 in, 1 out]
  n117 = call <vilib>:"DAQmx Clear Task.vi"("task in"=w17, "error in"=w18) -> ()  [unwired: 13 in, 1 out]
  n118 = Array Size(array=w40) -> (size(s)=→"size of saved output array":i32[])
  n119 = local read "TF_Params"() -> (w15:T3)
  n120 = case shown="True" "Save File?" {
    tunnel: w43 -> [_ w377]
    tunnel: w42 -> [_ w376]
    tunnel: w41 -> [_ w375]
    tunnel: w40 -> [_ w374]
    tunnel: w39 -> [_ w373]
    tunnel: "in:" -> [_ w372]
    tunnel: "string append to saved name" -> [_ w371]
    tunnel: "string 2" -> [_ w370]
    tunnel: ["" ("saved name:") w369] -> w30
    tunnel: w15 -> [_ w368]
    tunnel: w14 -> [_ w367]
    tunnel: w13 -> [_ w366]
    frame False {
    }
    frame True {
      n121 = call "Save_TF_Data.vi"("TF_Params"=w368, "Save Raw Data?"="Save Raw Data?", "Preamp Gain"="Preamp Gain", "in:"=w372, "TF Mag"=w376, "string"=w371, "string 2"=w370, "TF Phase"=w375, "data"=w374, "Freqs"=w377, "DividedCh2By"=w366, "Output Array"=w373, "DividedCh1By"=w367) -> ("saved name:"=w369:string)  [unwired: 2 in]
    }
  }
  "saved name:" <- w30
